vi "4Pi Objective Lock - EMBL-v1.vi"(7 "Calling VI Ref":refnum<vi>) -> ()   [LabVIEW 2016]
uses:
  <vilib>/Utility/miscctls.llb/LVPointTypeDef.ctl
  4Pi Objective Lock Type Defs/4Pi Obj Lock - Notifier Type.ctl
  4Pi Objective Lock Type Defs/4Pi Obj Lock - Actions.ctl
  <vilib>/vision/Image Controls.llb/IMAQ Image.ctl
  4Pi Objective Lock Type Defs/4Pi Obj Lock - Lock Settings.ctl
  Hardware Configuration/Hardware Configuration Controls/Device Type.ctl
  Hardware Configuration/Hardware Configuration Controls/Device Function.ctl
  4Pi Objective Lock Type Defs/4Pi Obj Lock - Camera Settings.ctl
  Device Library/Cameras/Camera Controls/Generic Camera ROI.ctl
  Device Library/Cameras/Camera Controls/Generic Camera Actions.ctl
  Device Library/Stages/Stages Controls/Stage Actions.ctl
  <vilib>/addons/control/pid/pid.llb/PID (DBL).vi
  <vilib>/addons/control/pid/pid.llb/PID (DBL Array).vi
  <vilib>/addons/control/pid/NI_PID_pid.lvlib
  <vilib>/vision/NI_Vision_Development_Module.lvlib
panel:
  out "dz (µm)":dbl format="%.2f"
  in  "Main Tab":T1(tab)
  out "Z Move":bool
  out "XY Move":bool
  out "Measured X Position (px)":dbl=1.0 format="%.3g"
  out "Measured Y Position (px)":dbl=1.0 format="%.3g"
  out "Measured sx/sy":dbl=1.0 format="%.3g"
  out "Target X Position (px)":dbl=1.0 format="%.3g"
  out "Target Y Position (px)":dbl=1.0 format="%.3g"
  out "Target sx/sy":dbl=1.0 format="%.3g"
  out "Z Axis Position (µm)":dbl=1.0 format="%.4g"
  out "Y Axis Position (µm)":dbl=1.0 format="%.2g"
  out "X Axis Position (µm)":dbl=1.0 format="%.2g"
  out "Z Target and Fit Value (µm)":T2(graph)
  in  "Start Lock":bool
  out "Y Target and Fit Position (µm)":T2(graph)
  out "X Target and Fit Position (µm)":T2(graph)
  in  "Restart Lock":bool
  out "Fit Error":bool
  out "Move Limit Error":bool
  out "Target Z (µm)":dbl=1.0 format="%.3g"
  out "Measured Z (µm)":dbl=1.0 format="%.3g"
  in  "pixel size (µm)":dbl=0.01
  in  "X Update Scale Factor":dbl=0.01
  in  "Y Update Scale Factor":dbl=0.01
  in  "Z Update Scale Factor":dbl=0.2
  in  "Sample Z Step No.":u32=2
  in  "Sample Z Step Size (µm)":dbl=2.0
  in  "Update Delay (ms)":i32=10
  in  "D (Derivative)":dbl
  in  "I (Integral)":dbl
  in  "P (Proportional)":dbl=2.0
  in  "Invert Z Axis":bool
  in  "XY Drift Threshold":dbl=0.05
  in  "Abort If Error":bool
  in  "Flip XY Axis":bool
  in  "Invert X Axis":bool=TRUE
  in  "Invert Y Axis":bool=TRUE
  in  "Z Stage Move Limit (µm)":dbl=5.0
  in  "Z Drift Threshold":dbl=0.05
  in  "XY Stage Move Limit (µm)":dbl=1.0
  in  "Frame Accumulations":u16=10
  in  "XY Correction Active":bool=TRUE
  in  "Z Correction Active":bool=TRUE
  in  "Set Camera ROI":bool
  in  "Save Lock Settings":bool
  in  "Quit":bool
  # "Z Drift Settings"
  # "Camera Setup"
  # "XY Drift Settings"
  # "PID Control Values"
  # "General Settings"
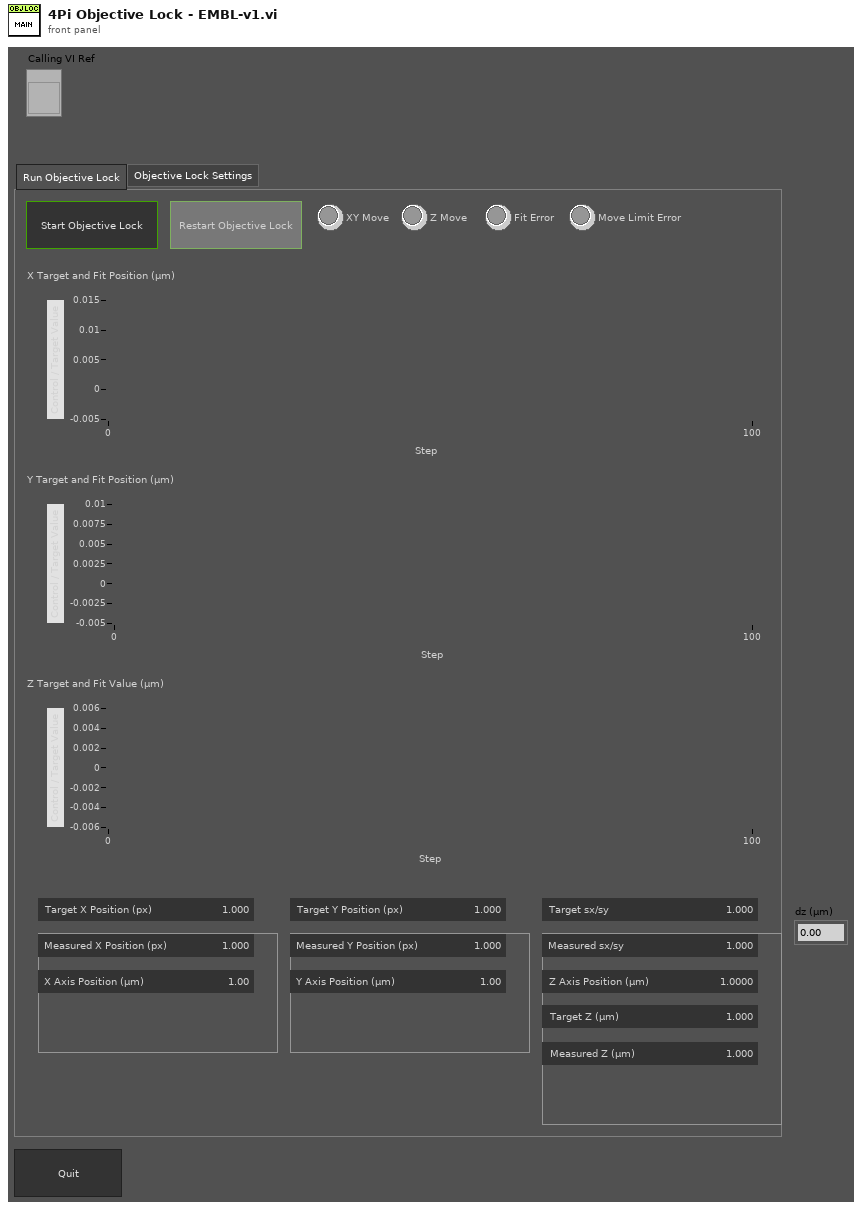
[diagram p1: front panel]
types:
  T1 = enum32{"Run Objective Lock", "Objective Lock Settings"}
  T2 = cluster{"Target 01":dbl, dbl, dbl, "Current 01":dbl, "Stage Pos":dbl}
  T3 = typedef "4Pi Obj Lock - Camera Settings.ctl" = cluster{"Exposure Time (s)":dbl, "H Offset":u16, "V Offset":u16, "H Width":u16, "V Width":u16}
  T4 = typedef "Device Function.ctl" = enum16{"Primary", "Secondary", "Overview", "Wide Field Drift Correction", "642 nm Excitation", "560 nm Excitation", "940 nm Excitation", "546 nm Excitation", "488 nm Excitation", "405 nm Excitation", "Objective Drift Correction", "4Pi Focus Lock", "4Pi Objective Lock", "Objective XY", "Objective Z", "Sample XY", "Sample Coarse Z", "Sample Z", "4Pi Lower", "4Pi Upper", "Mojo", "Adj Cavity", "Line Scanning", "Alert"}
  T5 = typedef "Device Type.ctl" = enum16{"AOTF", "Camera", "Deformable Mirror", "Laser", "Shutter", "Stage", "Waveform", "FPGA", "Email"}
  T6 = typedef "4Pi Obj Lock - Actions.ctl" = enum16{"Idle", "Start Lock", "Restart Lock", "Get Initial Position", "Get Target Z Position", "Get Ref Stack", "Cal Ref FFT", "Move To Init Z", "Get Current Z Position", "Get Current Position", "Check Drift", "Move XYZ", "Move XY", "Move Z", "Update Plots", "Delay", "Abort", "Exit Loop", "Quit"}
  T7 = typedef "4Pi Obj Lock - Lock Settings.ctl" = cluster{"Z Drift Threshold":dbl, "Z Stage Move Limit (µm)":dbl, "XY Drift Threshold":dbl, "XY Stage Move Limit (µm)":dbl, "Frame Accumulations":u16, "Abort If Error":bool, "Flip XY Axis":bool, "Invert X Axis":bool, "Invert Y Axis":bool, "Invert Z Axis":bool, "Z Correction Active":bool, "XY Correction Active":bool, "PID Values":dbl[], "Update Delay (ms)":i32, "Sample Z Step Size (µm)":dbl, "Sample Z Step No.":u32, "Z Update Scale Factor":dbl, "Y Update Scale Factor":dbl, "X Update Scale Factor":dbl}
  T8 = typedef "4Pi Obj Lock - Notifier Type.ctl" = cluster{"Actions":T6, "Z Drift Threshold":dbl, "Z Stage Move Limit (µm)":dbl, "XY Drift Threshold":dbl, "XY Stage Move Limit (µm)":dbl, "Frame Accumulations":u16, "Abort If Error":bool, "Z Correction Active":bool, "XY Correction Active":bool, "PID Values":dbl[], "Running?":bool, "Update Delay (ms)":i32, "Cur Image (SGL)":T9, "Ref Stack (SGL)":T9[], "Sample Z (µm)":dbl[], "Initial Z Position (µm)":dbl, "Z Step Size (µm)":dbl, "Z Step No.":u32, "Ref FFT Stack (CSG)":T9[], "CC Image (SGL) ":T9, "Tmp Image FFT (CSG)":T9[]}
  T9 = typedef "IMAQ Image.ctl" = refnum<image>
  T10 = enum16{"Always On", "Always Off", "Off While Running"}
  T11 = typedef "LVPointTypeDef.ctl" = cluster{"Horizontal":i16, "Vertical":i16}
  T12 = typedef "Image Type" = u32
  T13 = typedef "Generic Camera Actions.ctl" = enum16{"Status", "Live Preview", "Capture", "Abort", "Set Exposure Time (s)", "Get Exposure Time (s)", "Record Settings", "Set ROI", "Get ROI", "Defect Correction On/Off", "Cooler On/Off", "Fan On/Off", "Quit"}
  T14 = typedef "Generic Camera ROI.ctl" = cluster{"H_Offset":u16, "V_Offset":u16, "H_Width":u16, "V_Width":u16}
  T15 = typedef "Stage Actions.ctl" = enum16{"Get Position", "MVR", "MOVE", "HALT", "ONTARGET", "ERROR", "REFERENCE", "INIT", "VELOCITY", "STATUS", "EXIT", "HOME", "ZEROPOS", "NANOPOS", "ANALOG", "QUIT"}
  T16 = enum32{"Invalid", "Standard", "Closed", "Hidden", "Minimized", "Maximized"}
  T17 = cluster{"Target 01":dbl, dbl, dbl, "Current 01":dbl, "Stage Pos":dbl}[]
  T18 = typedef "Stage Status.ctl" = enum16{"Error", "Abort", "Busy", "On Target"}
  T19 = typedef "2D Gaussian - Best Fit Parameters.ctl" = cluster{"Amplitude":dbl, "X Position":dbl, "Y Position":dbl, "X Width":dbl, "Y Width":dbl, "Offset":dbl}
  T20 = cluster{"PID Values[0]":dbl, "PID Values[1]":dbl, "PID Values[2]":dbl}
  T21 = cluster{"PID Values[0]":dbl, "PID Values[1]":dbl, "PID Values[2]":dbl}[]
  T22 = typedef "LVRectTypeDef.ctl" = cluster{"Left":i16, "Top":i16, "Right":i16, "Bottom":i16}
  T23 = typedef "LVBoundsTypeDef.ctl" = cluster{"Width":u32, "Height":u32}
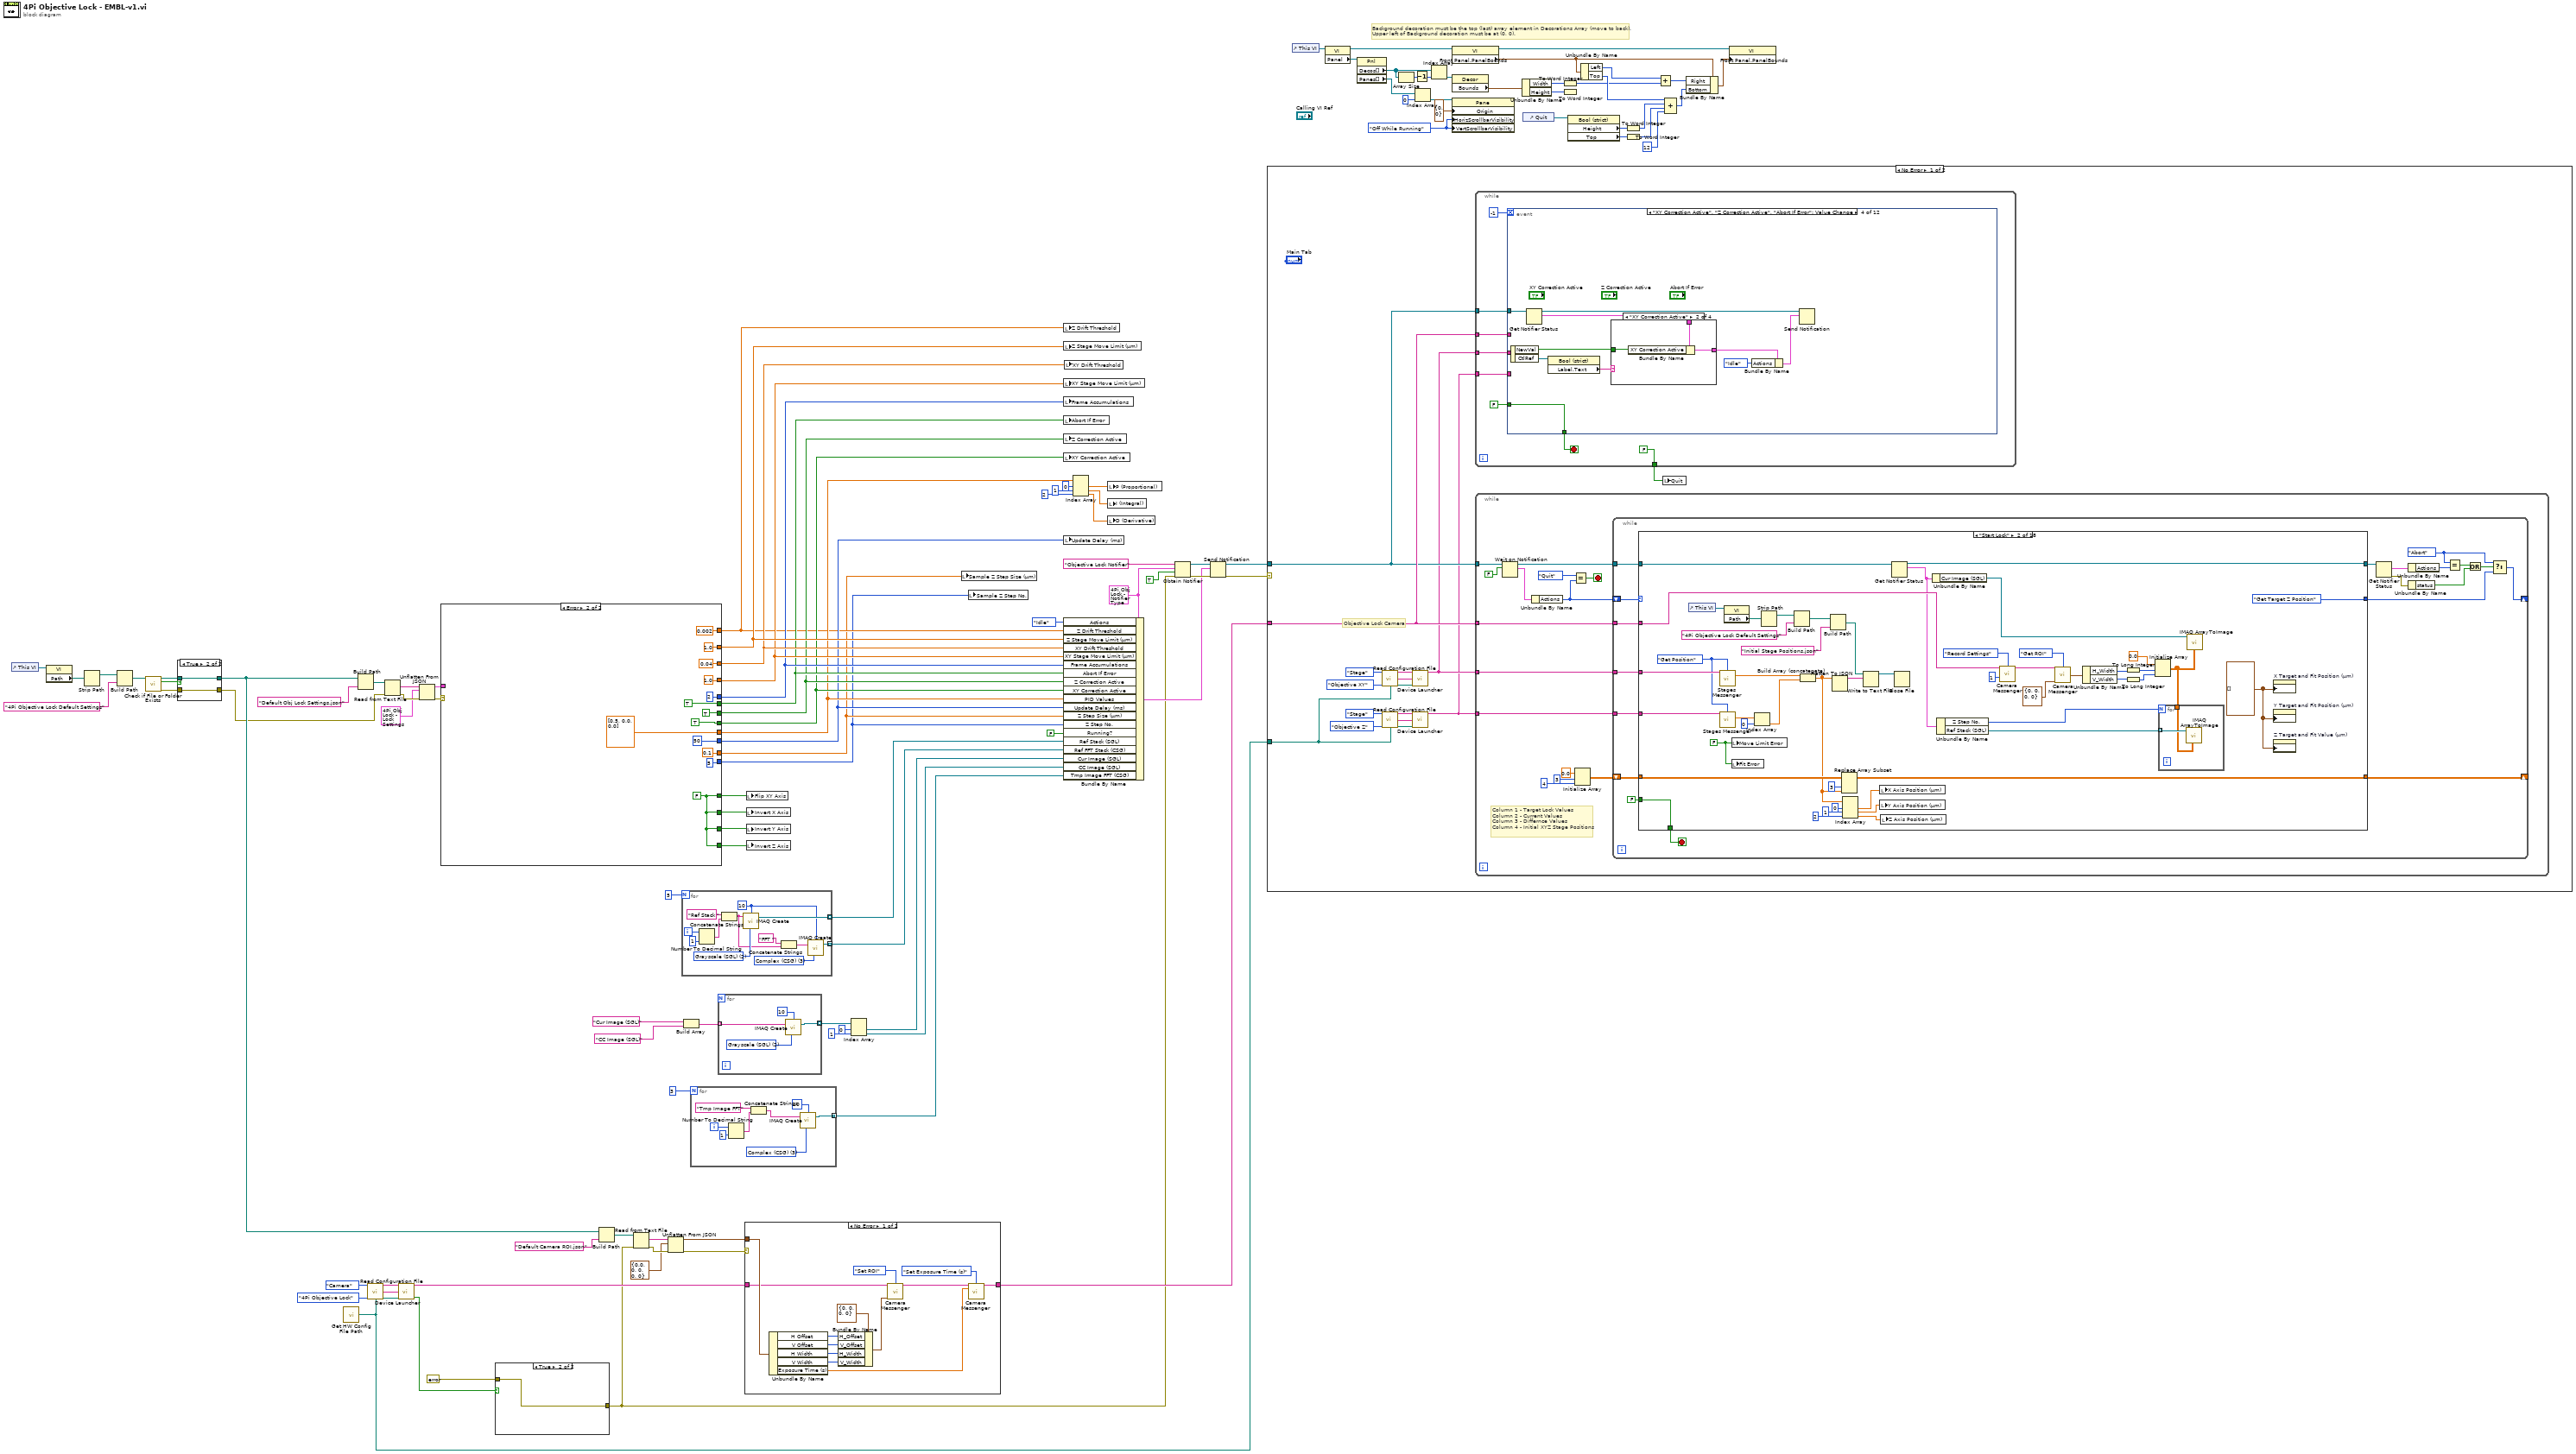
[diagram p0: block diagram]
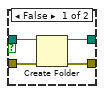
[diagram p2: hidden frame]
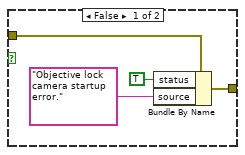
[diagram p3: hidden frame]
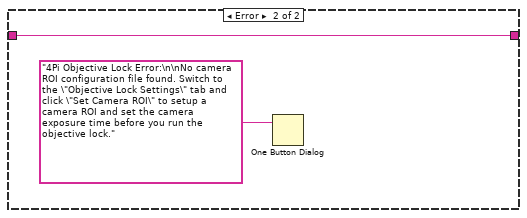
[diagram p4: hidden frame]
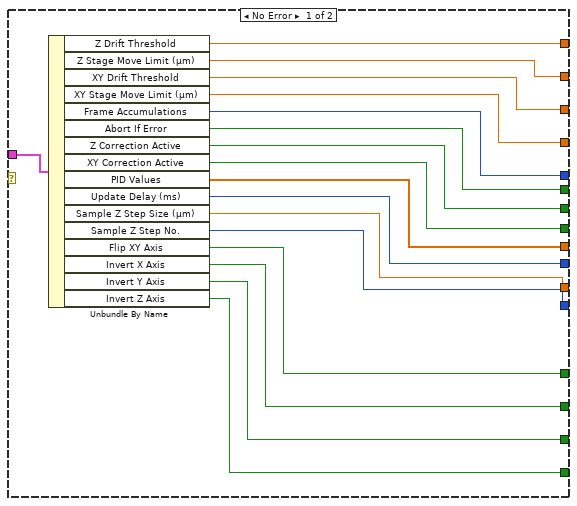
[diagram p5: hidden frame]
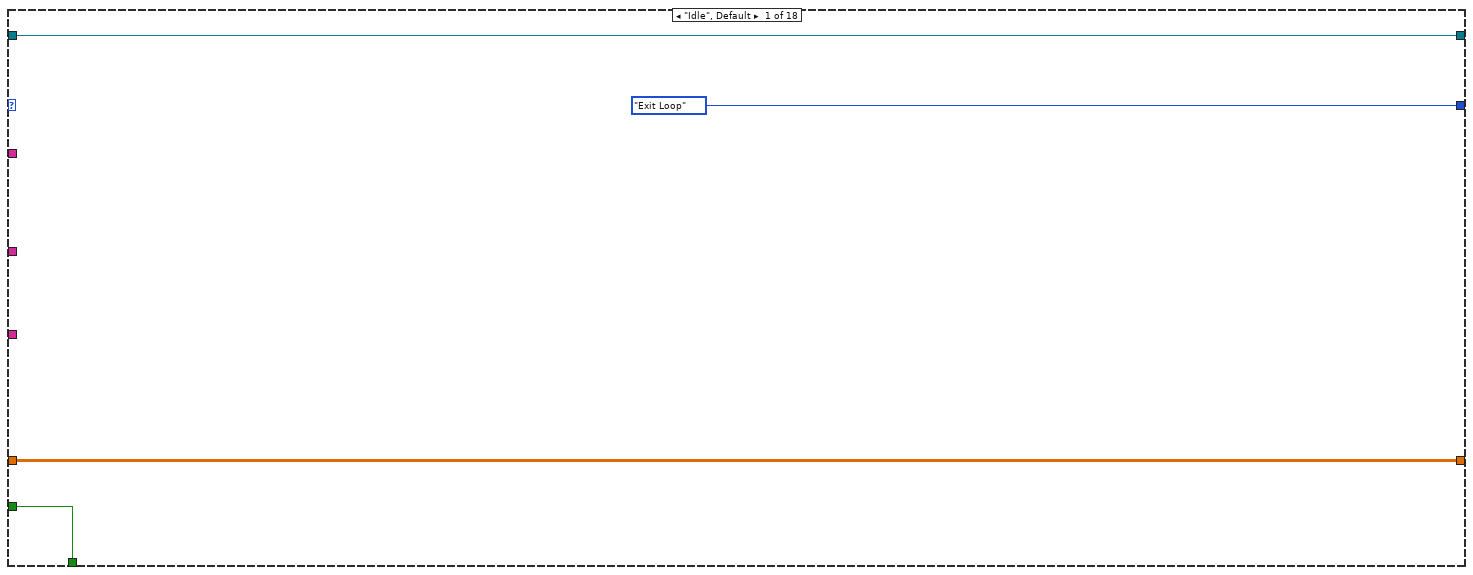
[diagram p6: hidden frame]
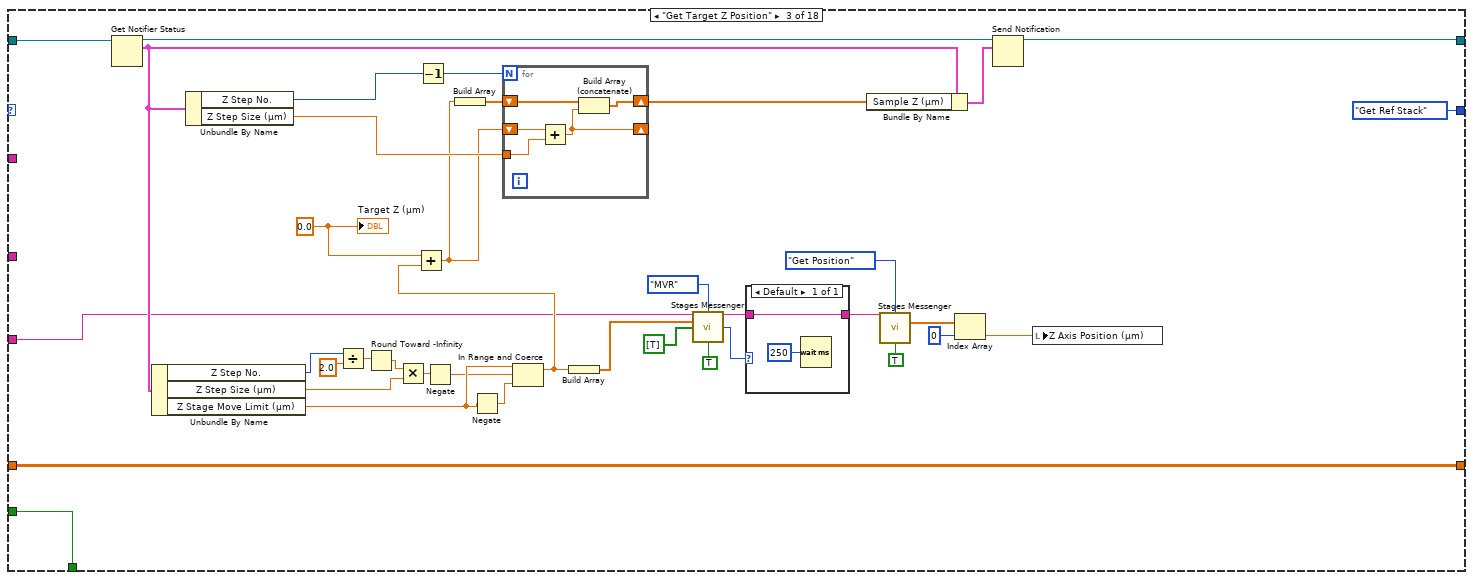
[diagram p7: hidden frame]
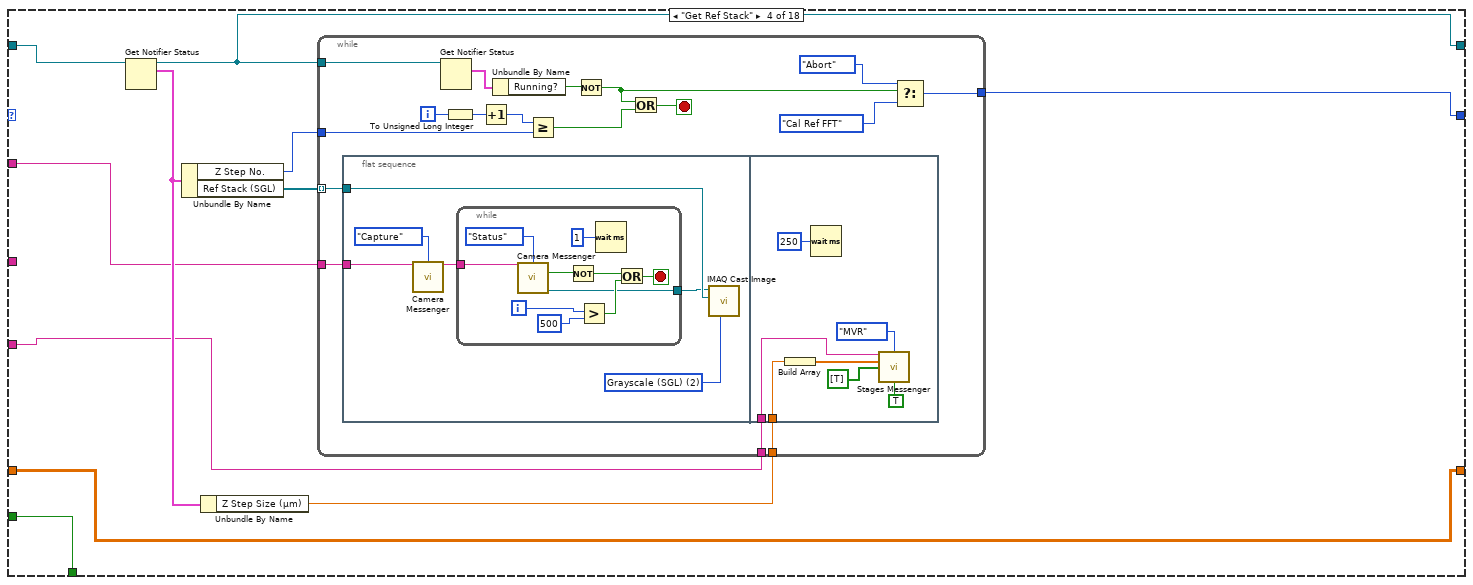
[diagram p8: hidden frame]
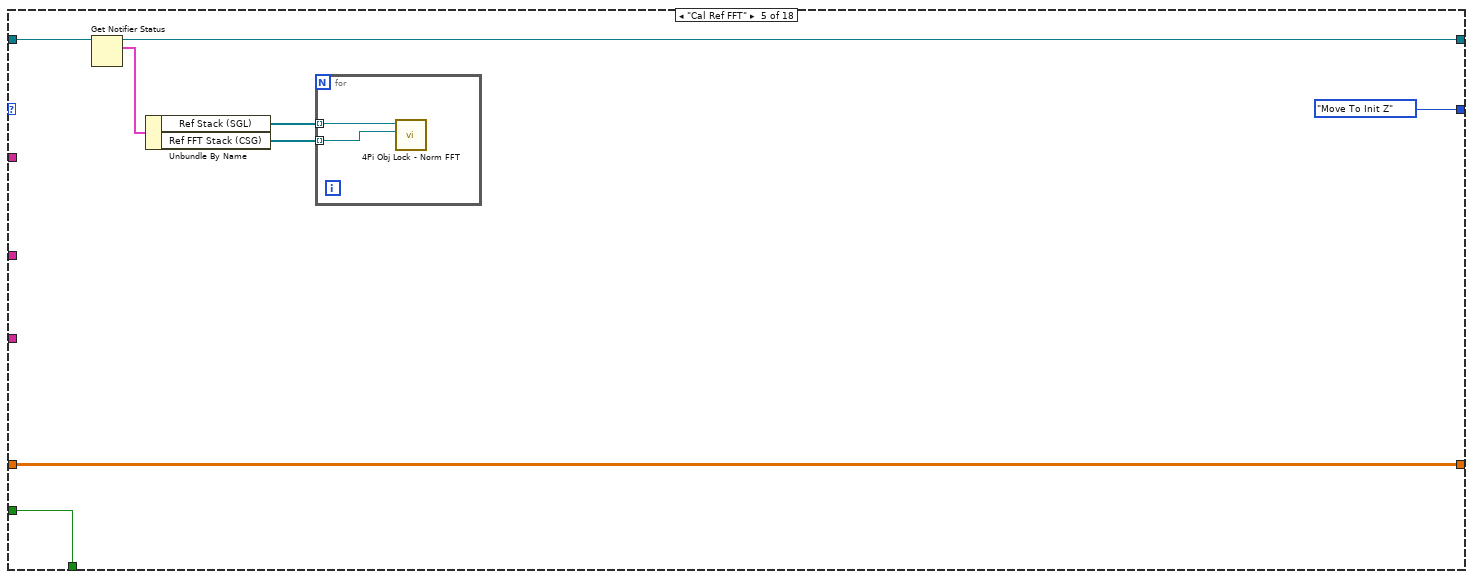
[diagram p9: hidden frame]
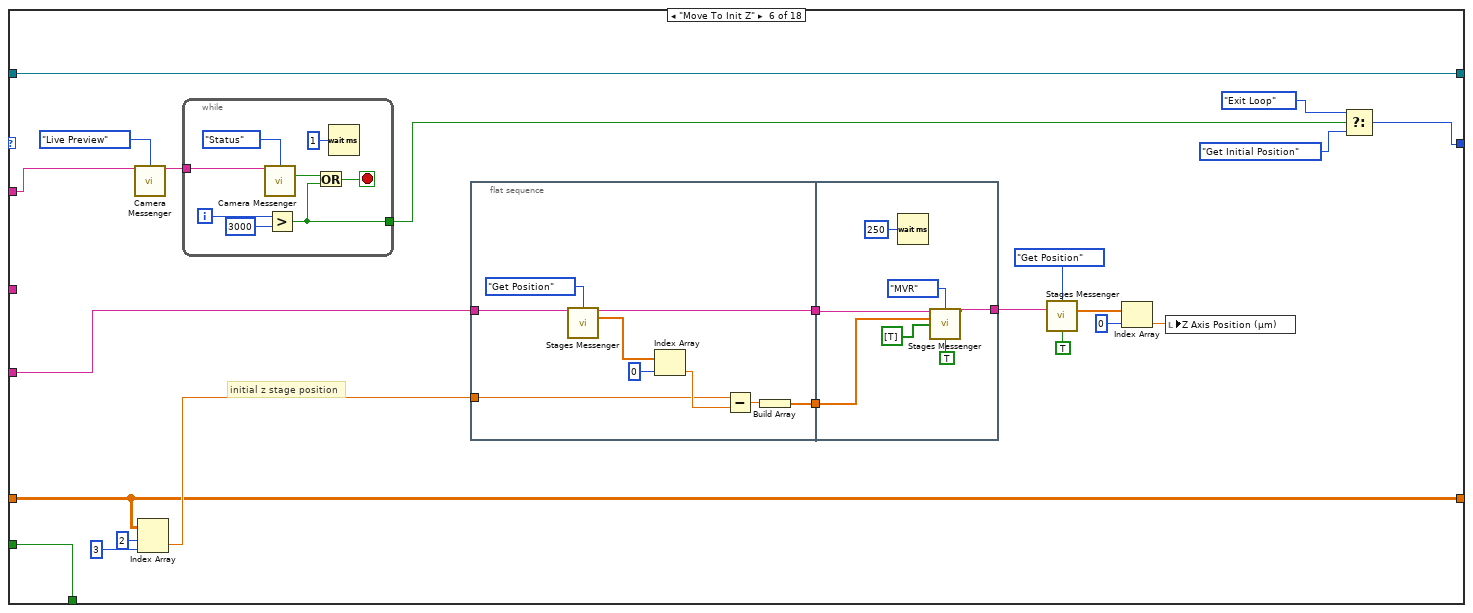
[diagram p10: hidden frame]
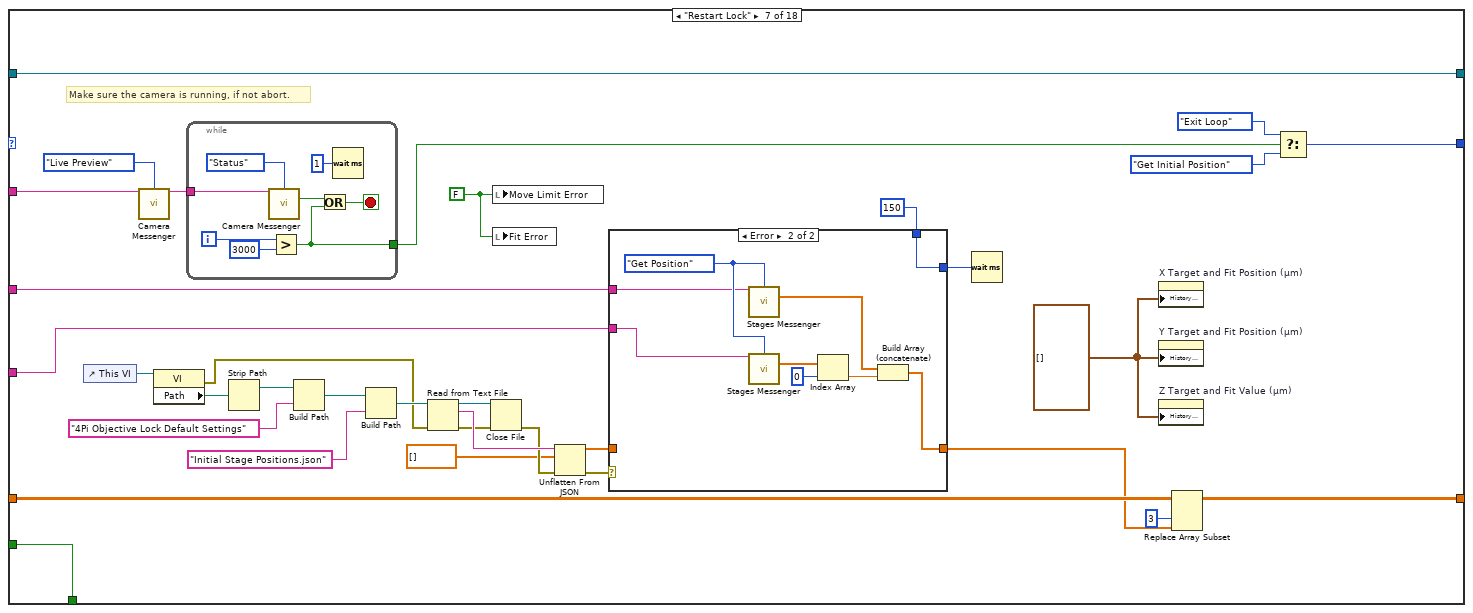
[diagram p11: hidden frame]
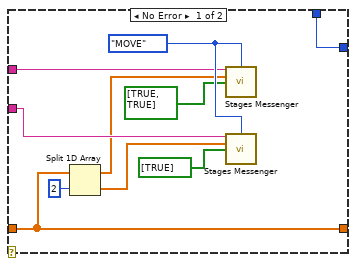
[diagram p12: hidden frame]
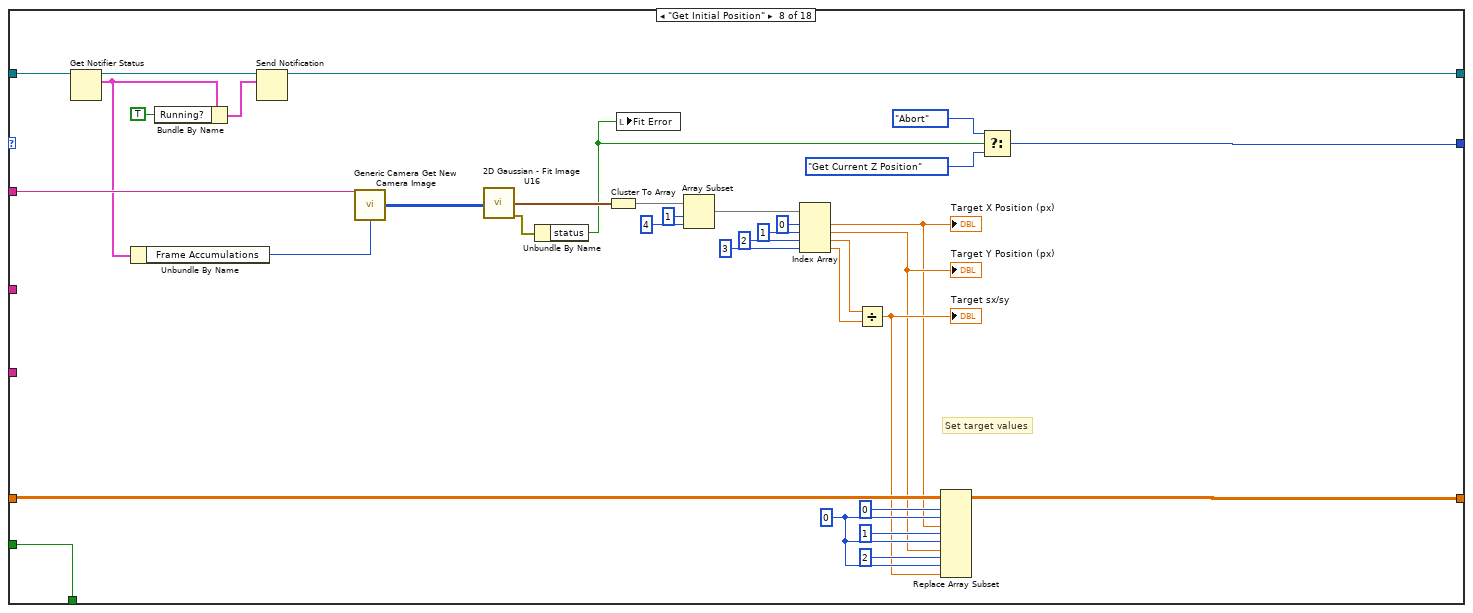
[diagram p13: hidden frame]
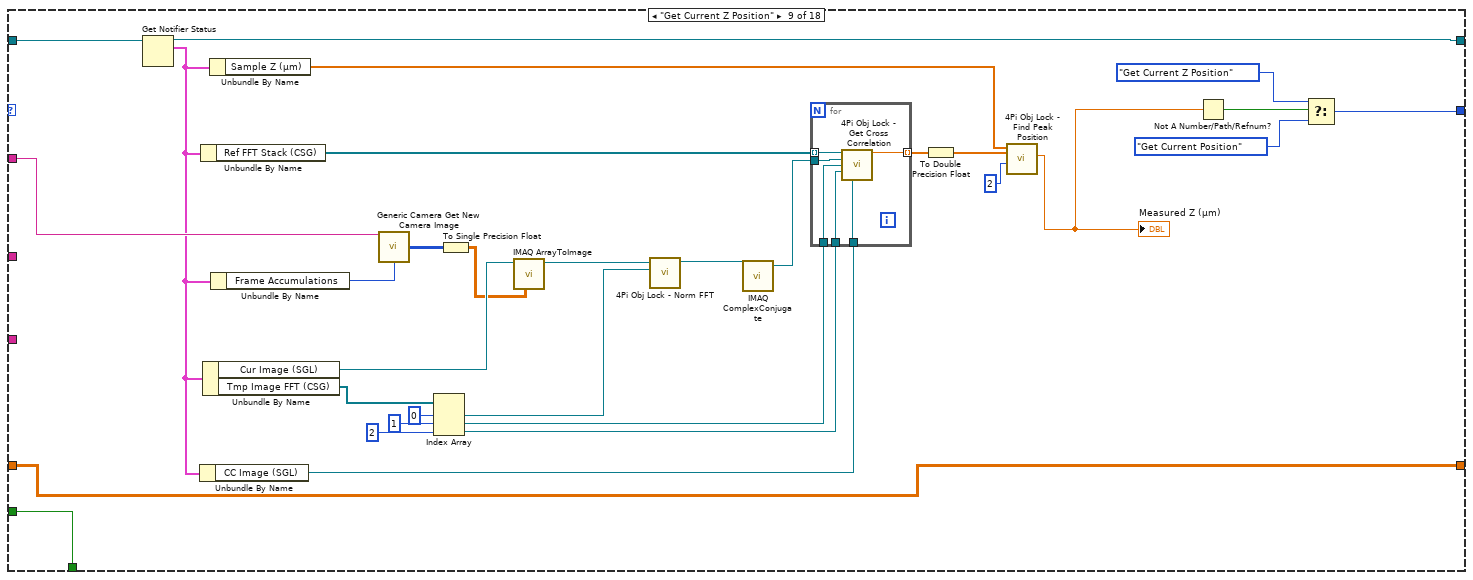
[diagram p14: hidden frame]
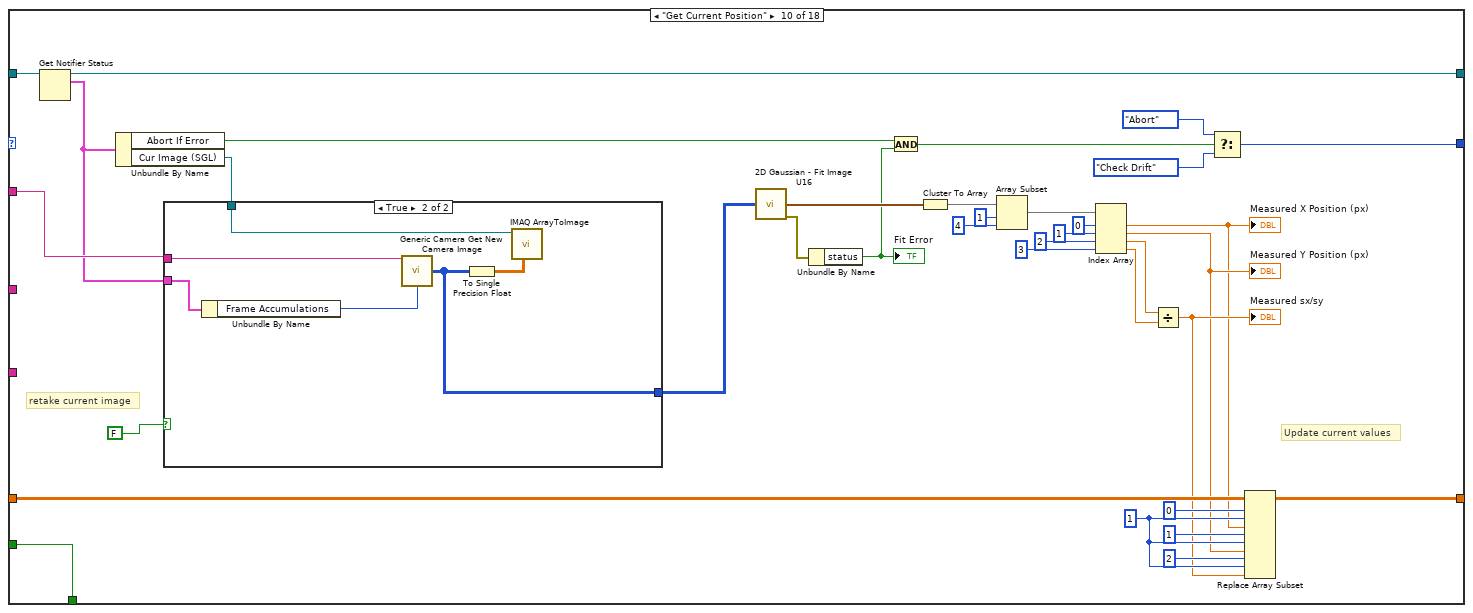
[diagram p15: hidden frame]
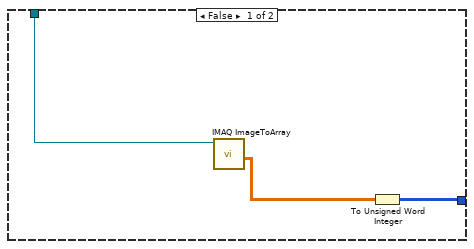
[diagram p16: hidden frame]
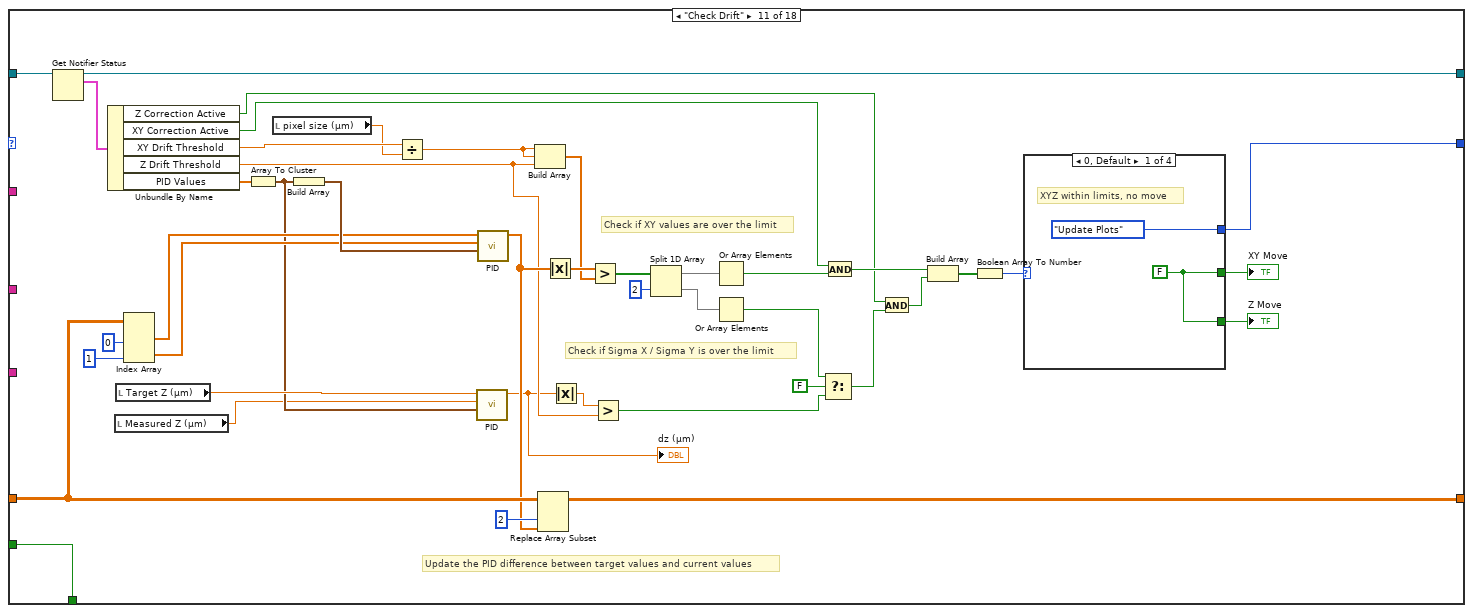
[diagram p17: hidden frame]
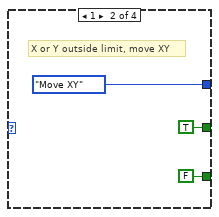
[diagram p18: hidden frame]
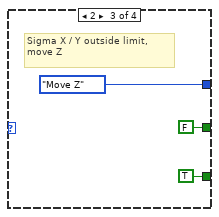
[diagram p19: hidden frame]
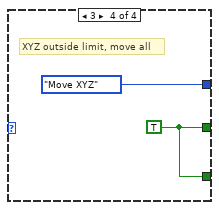
[diagram p20: hidden frame]
diagram:
  w75 = T8 {"Actions"=enum."Idle", "Z Drift Threshold"=0.05, "Z Stage Move Limit (µm)"=1.0, "XY Drift Threshold"=0.05, "XY Stage Move Limit (µm)"=1.0, "Frame Accumulations"=10, "Abort If Error"=FALSE, "Z Correction Active"=FALSE, "XY Correction Active"=FALSE, "PID Values"=[], "Running?"=FALSE, "Update Delay (ms)"=0, "Cur Image (SGL)"=refnum, "Ref Stack (SGL)"=[], "Sample Z (µm)"=[], "Initial Z Position (µm)"=0.0, "Z Step Size (µm)"=2.0, "Z Step No."=2, "Ref FFT Stack (CSG)"=[], "CC Image (SGL) "=refnum, "Tmp Image FFT (CSG)"=[]} ("4Pi Obj Lock")
  w92 = T10."Off While Running" ("Vertical Scrollbar Visibility")
  # "Background decoration must be the top (last) array element in Decorations Array (move to back).\nUpper left of Background decoration must be at (0, 0)."
  n1 = control-ref of="This VI"() -> (w63:refnum<vi>)
  n2 = property class="VI"(reference=w63) -> ("Path"=w45:path)  [unwired: 1 in, 2 out]
  n3 = Strip Path(path=w45) -> (stripped path=w44:path)  [unwired: 1 out]
  n4 = Build Path(base path=w44, name or relative path="4Pi Objective Lock Default Settings") -> (appended path=w21:path)
  n5 = call <vilib>:"Check if File or Folder Exists.vi"("path"=w21) -> ("error out"=w17:errorcluster, "file or folder exists?"=w20:bool, "dup path"=w19:path)  [unwired: 8 in]
  n6 = case shown="True" w20 {
    tunnel: w19 -> [w113 w115]
    tunnel: [w112 w115] -> w18
    tunnel: w17 -> [w111 w114]
    tunnel: [w110 w114] -> w16
    frame False {
      n7 = Create Folder(path (use dialog)=w113, error in=w111) -> (created path=w112:path, error out=w110:errorcluster)  [unwired: 1 in, 1 out]
    }
    frame True {
    }
  }
  n8 = call "Get HW Config File Path.vi"() -> ("File Path"=w53:path)  [unwired: 14 in, 1 out]
  n9 = Build Path(base path=w18, name or relative path="Default Obj Lock Settings.json") -> (appended path=w72:path)
  n10 = call "Read Configuration File.vi"("Device Type"=Device_Type."Camera", "Device Function"=Device_Function."4Pi Objective Lock", "Config File Path"=w53) -> ("Unique Notifier Name"=w60:string, "Device Ports/IDs/Channels"=w62:string[], "Device Engine Path"=w61:path)  [unwired: 9 in, 1 out]
  n11 = Read from Text File(file (use dialog)=w72, error in=w16) -> (text=w71:string, error out=w70:errorcluster)  [unwired: 2 in, 2 out]
  n12 = call "Device Launcher.vi"("Notifier Name"=w60, "Device Ports/IDs/Channels"=w62, "Device Engine Path"=w61) -> ("Notifier Name"=w51:string, "Running?"=w57:bool)  [unwired: 11 in]
  n13 = Unflatten From JSON(JSON string=w71, type and defaults=T7 {"Z Drift Threshold"=0.05, "Z Stage Move Limit (µm)"=1.0, "XY Drift Threshold"=0.05, "XY Stage Move Limit (µm)"=1.0, "Frame Accumulations"=10, "Abort If Error"=FALSE, "Flip XY Axis"=FALSE, "Invert X Axis"=FALSE, "Invert Y Axis"=FALSE, "Invert Z Axis"=FALSE, "Z Correction Active"=TRUE, "XY Correction Active"=TRUE, "PID Values"=[], "Update Delay (ms)"=0, "Sample Z Step Size (µm)"=2.0, "Sample Z Step No."=2, "Z Update Scale Factor"=2.0, "Y Update Scale Factor"=2.0, "X Update Scale Factor"=2.0} ("Lock Settings"), error in (no error)=w70) -> (value=w67:T7, error out=w68:errorcluster)  [unwired: 4 in]
  n14 = case shown="Error" w68 {
    tunnel: [w131 0.002 ("Z Drift Threshold")] -> w22
    tunnel: [w130 1.0 ("Z Stage Move Limit (µm)")] -> w37
    tunnel: [w128 0.04 ("XY Drift Threshold")] -> w36
    tunnel: [w129 1.0 ("XY Stage Move Limit (µm)")] -> w35
    tunnel: [w127 u16 2 ("Frame Accumulations")] -> w34
    tunnel: [w126 TRUE ("Abort If Error")] -> w33
    tunnel: w67 -> [w132 _]
    tunnel: [w125 TRUE ("Z Correction Active")] -> w32
    tunnel: [w124 TRUE ("XY Correction Active")] -> w31
    tunnel: [w123 dbl[] [0.5, 0.0, 0.0] ("PID Values")] -> w30
    tunnel: [w122 u16 50 ("Update Delay (ms)")] -> w23
    tunnel: [w121 w135] -> w39
    tunnel: [w120 w135] -> w40
    tunnel: [w119 w135] -> w41
    tunnel: [w118 w135] -> w42
    tunnel: [w117 0.1 ("Sample Z Step Size (µm)")] -> w2
    tunnel: [w116 u32 5 ("Sample Z Step No.")] -> w1
    frame No Error {
      n15 = Unbundle By Name(w132) -> ("Z Drift Threshold"=w131:dbl, "Z Stage Move Limit (µm)"=w130:dbl, "XY Drift Threshold"=w128:dbl, "XY Stage Move Limit (µm)"=w129:dbl, "Frame Accumulations"=w127:u16, "Abort If Error"=w126:bool, "Z Correction Active"=w125:bool, "XY Correction Active"=w124:bool, "PID Values"=w123:dbl[], "Update Delay (ms)"=w122:i32, "Sample Z Step Size (µm)"=w117:dbl, "Sample Z Step No."=w116:u32, "Flip XY Axis"=w118:bool, "Invert X Axis"=w119:bool, "Invert Y Axis"=w120:bool, "Invert Z Axis"=w121:bool)
    }
    frame Error {
      w135 = FALSE ("Flip XY Axis")
    }
  }
  n16 = case shown="True" w57 {
    tunnel: errorcluster {"status"=FALSE, "code"=0, "source"=""} ("Error") -> [w149 w150]
    tunnel: [w146 w150] -> w43
    frame False {
      n17 = Bundle By Name(cluster=w149, "status"=TRUE, "source"="Objective lock camera startup error." ("name or relative path")) -> (w146:errorcluster)
    }
    frame True {
    }
  }
  n18 = Build Path(base path=w18, name or relative path="Default Camera ROI.json") -> (appended path=w47:path)
  n19 = Read from Text File(file (use dialog)=w47, error in=w43) -> (text=w65:string, error out=w64:errorcluster)  [unwired: 2 in, 2 out]
  n20 = Unflatten From JSON(JSON string=w65, type and defaults=T3 {"Exposure Time (s)"=0.0, "H Offset"=0, "V Offset"=0, "H Width"=0, "V Width"=0} ("Camera Settings"), error in (no error)=w64) -> (value=w50:T3, error out=w55:errorcluster)  [unwired: 4 in]
  n21 = for {
    N: 5 -> [_]
    tunnel: [w162] -> w14 mode=indexing
    tunnel: [w151] -> w13 mode=indexing
    i -> [w161]
    w156 = T12 3 items=["Grayscale (U8)", "Grayscale (I16)", "Grayscale (SGL)", "Complex (CSG)", "RGB (U32)", "HSL (U32)", "RGB (U64)", "Grayscale (U16)"] ("Image Type")
    w157 = T12 2 items=["Grayscale (U8)", "Grayscale (I16)", "Grayscale (SGL)", "Complex (CSG)", "RGB (U32)", "HSL (U32)", "RGB (U64)", "Grayscale (U16)"] ("Image Type")
    w153 = 10 ("Border Size")
    n22 = Number To Decimal String(number=w161, width (-)=i16 1) -> (decimal integer string=w159:string)
    n23 = Concatenate Strings("Ref Stack " ("string"), w159) -> (w152:string)
    n24 = call "IMAQ Create"("Border Size"=w153, "Image Name"=w152, "Image Type"=w157) -> ("New Image"=w162:T9)  [unwired: 2 in, 1 out]
    n25 = Concatenate Strings("FFT " ("string"), w152) -> (w155:string)
    n26 = call "IMAQ Create"("Border Size"=w153, "Image Name"=w155, "Image Type"=w156) -> ("New Image"=w151:T9)  [unwired: 2 in, 1 out]
  }
  n27 = Build Array("Cur Image (SGL)" ("Image Name"), "CC Image (SGL)" ("Image Name")) -> (w8:string[])
  n28 = for {
    N: 3 -> [_]
    tunnel: [w168] -> w3 mode=indexing
    i -> [w164]
    w169 = T12 3 items=["Grayscale (U8)", "Grayscale (I16)", "Grayscale (SGL)", "Complex (CSG)", "RGB (U32)", "HSL (U32)", "RGB (U64)", "Grayscale (U16)"] ("Image Type")
    n29 = Number To Decimal String(number=w164, width (-)=i16 1) -> (decimal integer string=w167:string)
    n30 = Concatenate Strings("Tmp Image FFT" ("Image Name"), w167) -> (w163:string)
    n31 = call "IMAQ Create"("Border Size"=10, "Image Name"=w163, "Image Type"=w169) -> ("New Image"=w168:T9)  [unwired: 2 in, 1 out]
  }
  n32 = for {
    tunnel: w8 -> [w172] mode=indexing
    tunnel: [w171] -> w7 mode=indexing
    w173 = T12 2 items=["Grayscale (U8)", "Grayscale (I16)", "Grayscale (SGL)", "Complex (CSG)", "RGB (U32)", "HSL (U32)", "RGB (U64)", "Grayscale (U16)"] ("Image Type")
    n33 = call "IMAQ Create"("Border Size"=10, "Image Name"=w172, "Image Type"=w173) -> ("New Image"=w171:T9)  [unwired: 2 in, 1 out]
  }
  n34 = case shown="No Error" w55 {
    tunnel: w51 -> [w178 w189]
    tunnel: w50 -> [w187 _]
    tunnel: [w175 w189] -> w49
    frame No Error {
      n35 = Unbundle By Name(w187) -> ("H Offset"=w182:u16, "V Offset"=w183:u16, "H Width"=w184:u16, "V Width"=w185:u16, "Exposure Time (s)"=w177:dbl)
      n36 = Bundle By Name(cluster=T14 {"H_Offset"=0, "V_Offset"=0, "H_Width"=0, "V_Width"=0} ("General Camera ROI"), "H_Offset"=w182, "V_Offset"=w183, "H_Width"=w184, "V_Width"=w185) -> (w181:T14)
      n37 = call "Camera Messenger.vi"("Notifier Name"=w178, "General Camera Actions"=Generic_Camera_Actions."Set ROI", "Camera ROI"=w181) -> ("Notifier Name Dup"=w176:string)  [unwired: 7 in, 5 out]
      n38 = call "Camera Messenger.vi"("Notifier Name"=w176, "General Camera Actions"=Generic_Camera_Actions."Set Exposure Time (s)", "Exposure Time (s)"=w177) -> ("Notifier Name Dup"=w175:string)  [unwired: 7 in, 5 out]
    }
    frame Error {
      n39 = One Button Dialog(message="4Pi Objective Lock Error:\n\nNo camera ROI configuration file found. Switch to the \"Objective Lock Settings\" tab and click \"Set Camera ROI\" to setup a camera ROI and set the camera exposure time before you run the objective lock.") -> ()  [unwired: 1 in, 1 out]
    }
  }
  n40 = local write "Flip XY Axis"(w42) -> ()
  n41 = local write "Invert X Axis"(w41) -> ()
  n42 = local write "Invert Y Axis"(w40) -> ()
  n43 = local write "Invert Z Axis"(w39) -> ()
  n44 = Index Array(array=w7, index #1=0 ("index"), index #2=1 ("index")) -> (element #1=w6:T9, element #2=w5:T9)
  n45 = local write "Sample Z Step Size (µm)"(w2) -> ()
  n46 = local write "Sample Z Step No."(w1) -> ()
  n47 = Bundle By Name(cluster=w75, "Actions"=4Pi_Obj_Lock_-_Actions."Idle", "Z Drift Threshold"=w22, "Z Stage Move Limit (µm)"=w37, "XY Drift Threshold"=w36, "XY Stage Move Limit (µm)"=w35, "Frame Accumulations"=w34, "Abort If Error"=w33, "Z Correction Active"=w32, "XY Correction Active"=w31, "PID Values"=w30, "Update Delay (ms)"=w23, "Z Step Size (µm)"=w2, "Z Step No."=w1, "Running?"=FALSE ("Obj Lock Active?"), "Ref Stack (SGL)"=w14, "Ref FFT Stack (CSG)"=w13, "Cur Image (SGL)"=w6, "CC Image (SGL)"=w5, "Tmp Image FFT (CSG)"=w3) -> (w74:T8)
  n48 = local write "Z Drift Threshold"(w22) -> ()
  n49 = local write "Z Stage Move Limit (µm)"(w37) -> ()
  n50 = local write "XY Stage Move Limit (µm)"(w35) -> ()
  n51 = local write "Frame Accumulations"(w34) -> ()
  n52 = local write "Abort If Error"(w33) -> ()
  n53 = local write "Z Correction Active"(w32) -> ()
  n54 = local write "XY Correction Active"(w31) -> ()
  n55 = local write "Update Delay (ms)"(w23) -> ()
  n56 = local write "XY Drift Threshold"(w36) -> ()
  n57 = Index Array(array=w30, index #1=0 ("index"), index #2=1 ("index"), index #3=2 ("index")) -> (element #1=w26:dbl, element #2=w24:dbl, element #3=w25:dbl)
  n58 = local write "P (Proportional)"(w26) -> ()
  n59 = local write "I (Integral)"(w24) -> ()
  n60 = local write "D (Derivative)"(w25) -> ()
  n61 = Obtain Notifier(name (unnamed)="Objective Lock Notifier", notification data type=w75, create if not found? (T)=TRUE, error in (no error)=w43) -> (notifier out=w77:refnum<notifier>, error out=w78:errorcluster)  [unwired: 1 out]
  n62 = Send Notification(notification=w74, notifier=w77, error in (no error)=w78) -> (notifier out=w76:refnum<notifier>, error out=w54:errorcluster)
  n63 = case shown="No Error" w54 {
    tunnel: w53 -> [w194 _]
    tunnel: w76 -> [w192 _]
    tunnel: w49 -> [w193 _]
    frame No Error {
      # "Objective Lock Camera"
      n64 = call "Read Configuration File.vi"("Device Type"=Device_Type."Stage", "Device Function"=Device_Function."Objective XY", "Config File Path"=w194) -> ("Unique Notifier Name"=w202:string, "Device Ports/IDs/Channels"=w200:string[], "Device Engine Path"=w201:path)  [unwired: 9 in, 1 out]
      n65 = call "Read Configuration File.vi"("Device Type"=Device_Type."Stage", "Device Function"=Device_Function."Objective Z", "Config File Path"=w194) -> ("Unique Notifier Name"=w197:string, "Device Ports/IDs/Channels"=w199:string[], "Device Engine Path"=w198:path)  [unwired: 9 in, 1 out]
      n66 = call "Device Launcher.vi"("Notifier Name"=w202, "Device Ports/IDs/Channels"=w200, "Device Engine Path"=w201) -> ("Notifier Name"=w191:string)  [unwired: 11 in, 1 out]
      n67 = call "Device Launcher.vi"("Notifier Name"=w197, "Device Ports/IDs/Channels"=w199, "Device Engine Path"=w198) -> ("Notifier Name"=w190:string)  [unwired: 11 in, 1 out]
      n68 = while {
        tunnel: [FALSE] -> w205
        tunnel: w193 -> [w898]
        tunnel: w192 -> [w897]
        tunnel: w191 -> [w896]
        tunnel: w190 -> [w895]
        stop <- w900 stop-if-true
        n69 = event shown="[3] \"XY Correction Active\", \"Z Correction Active\", \"Abort If Error\": Value Change" {
          selector: _ -> [_ _ _ _ _ _ _ _ _ _ _ _]
          dyn-events: _ -> [_ _ _ _ _ _ _ _ _ _ _ _]
          timeout: -1 -> [_ _ _ _ _ _ _ _ _ _ _ _]
          tunnel: FALSE -> [w903 w907 w910 w920 w940 w975 w1002 w1009 w1038 w1048 w1055 _]
          tunnel: [w903 w907 w910 w920 w940 w975 w1002 w1009 w1038 w1048 w1055 w1065] -> w900
          tunnel: w898 -> [_ _ w909 _ _ _ _ _ _ _ _ _]
          tunnel: w897 -> [_ _ _ w919 w937 w978 w1001 w1008 w1037 w1047 w1054 w1060]
          tunnel: w896 -> [_ _ _ _ _ _ _ _ _ _ _ _]
          tunnel: w895 -> [_ _ _ _ _ _ _ _ _ _ _ _]
          event Timeout {
            n70 = event-data() -> ()  [unwired: 1 in, 1 out]
          }
          event Application Instance Close? {
            n71 = event-data() -> ()  [unwired: 1 in, 1 out]
            n72 = control-ref of="This VI"() -> (w904:refnum<vi>)
            n73 = invoke class="VI" method="FP.Open"(reference=w904, "Activate"=TRUE ("Activate?"), "State"=T16."Standard") -> ()  [unwired: 2 in, 5 out]
            n74 = event-data("Discard?"=TRUE) -> ()  [unwired: 1 in, 1 out]
          }
          event "Set Camera ROI": Value Change {
            n75 = event-data() -> ()  [unwired: 1 in, 2 out]
            n76 = call "4Pi Obj Lock - Setup Camera.vi"("Camera Notifier Name"=w909) -> ()  [unwired: 14 in, 1 out]
          }
          event "XY Correction Active", "Z Correction Active", "Abort If Error": Value Change {
            n77 = event-data() -> ("NewVal"=w915:bool, "CtlRef"=w918:refnum<vi>)  [unwired: 1 in]
            n78 = Get Notifier Status(notifier=w919) -> (notifier out=w917:refnum<notifier>, current notification=w914:T8)  [unwired: 1 in, 3 out]
            n79 = property class="Bool (strict)"(reference=w918) -> ("Label.Text"=w916:string)  [unwired: 1 in, 2 out]
            n80 = case shown="\"XY Correction Active\"" w916 {
              tunnel: w915 -> [_ w923 w926 w929]
              tunnel: w914 -> [w921 w924 w927 w930]
              tunnel: [w921 w922 w925 w928] -> w913
              frame Default {
              }
              frame "XY Correction Active" {
                n81 = Bundle By Name(cluster=w924, "XY Correction Active"=w923) -> (w922:T8)
              }
              frame "Z Correction Active" {
                n82 = Bundle By Name(cluster=w927, "Z Correction Active"=w926) -> (w925:T8)
              }
              frame "Abort If Error" {
                n83 = Bundle By Name(cluster=w930, "Abort If Error"=w929) -> (w928:T8)
              }
            }
            n84 = Bundle By Name(cluster=w913, "Actions"=4Pi_Obj_Lock_-_Actions."Idle") -> (w911:T8)
            n85 = Send Notification(notification=w911, notifier=w917) -> ()  [unwired: 1 in, 2 out]
          }
          event "Z Drift Threshold", "Z Stage Move Limit (µm)", "XY Drift Threshold", "XY Stage Move Limit (µm)", "P (Proportional)", "I (Integral)", "D (Derivative)", "Sample Z Step Size (µm)": Value Change {
            n86 = event-data() -> ("NewVal"=w935:dbl, "CtlRef"=w936:refnum<vi>)  [unwired: 1 in]
            n87 = Get Notifier Status(notifier=w937) -> (notifier out=w934:refnum<notifier>, current notification=w938:T8)  [unwired: 1 in, 3 out]
            n88 = property class="DigNum (strict)"(reference=w936) -> ("Label.Text"=w939:string)  [unwired: 1 in, 2 out]
            n89 = case shown="\"Sample Z Step Size (µm)\"" w939 {
              tunnel: w935 -> [_ w943 w946 w949 w952 w957 w963 w969 w973]
              tunnel: w938 -> [w941 w944 w947 w950 w953 w956 w962 w968 w974]
              tunnel: [w941 w942 w945 w948 w951 w954 w960 w966 w972] -> w932
              frame Default {
              }
              frame "Z Drift Threshold" {
                n90 = Bundle By Name(cluster=w944, "Z Drift Threshold"=w943) -> (w942:T8)
              }
              frame "Z Stage Move Limit (µm)" {
                n91 = Bundle By Name(cluster=w947, "Z Stage Move Limit (µm)"=w946) -> (w945:T8)
              }
              frame "XY Drift Threshold" {
                n92 = Bundle By Name(cluster=w950, "XY Drift Threshold"=w949) -> (w948:T8)
              }
              frame "XY Stage Move Limit (µm)" {
                n93 = Bundle By Name(cluster=w953, "XY Stage Move Limit (µm)"=w952) -> (w951:T8)
              }
              frame "P (Proportional)" {
                n94 = Unbundle By Name(w956) -> ("PID Values"=w959:dbl[])
                n95 = Replace Array Subset(array=w959, new element=w957, index=0) -> (w955:dbl[])
                n96 = Bundle By Name(cluster=w956, "PID Values"=w955) -> (w954:T8)
              }
              frame "I (Integral)" {
                n97 = Unbundle By Name(w962) -> ("PID Values"=w965:dbl[])
                n98 = Replace Array Subset(array=w965, new element=w963, index=1) -> (w961:dbl[])
                n99 = Bundle By Name(cluster=w962, "PID Values"=w961) -> (w960:T8)
              }
              frame "D (Derivative)" {
                n100 = Unbundle By Name(w968) -> ("PID Values"=w971:dbl[])
                n101 = Replace Array Subset(array=w971, new element=w969, index=2) -> (w967:dbl[])
                n102 = Bundle By Name(cluster=w968, "PID Values"=w967) -> (w966:T8)
              }
              frame "Sample Z Step Size (µm)" {
                n103 = Bundle By Name(cluster=w974, "Z Step Size (µm)"=w973) -> (w972:T8)
              }
            }
            n104 = Bundle By Name(cluster=w932, "Actions"=4Pi_Obj_Lock_-_Actions."Idle") -> (w931:T8)
            n105 = Send Notification(notification=w931, notifier=w934) -> ()  [unwired: 1 in, 2 out]
          }
          event "Sample Z Step No.": Value Change {
            n106 = event-data() -> ("NewVal"=w976:u32)  [unwired: 1 in]
            n107 = for {
              N: w976 -> [_]
              tunnel: [w995] -> w980 mode=indexing
              tunnel: [w984] -> w979 mode=indexing
              i -> [w994]
              w985 = T12 3 items=["Grayscale (U8)", "Grayscale (I16)", "Grayscale (SGL)", "Complex (CSG)", "RGB (U32)", "HSL (U32)", "RGB (U64)", "Grayscale (U16)"] ("Image Type")
              w990 = T12 2 items=["Grayscale (U8)", "Grayscale (I16)", "Grayscale (SGL)", "Complex (CSG)", "RGB (U32)", "HSL (U32)", "RGB (U64)", "Grayscale (U16)"] ("Image Type")
              w986 = 10 ("Border Size")
              n108 = Number To Decimal String(number=w994, width (-)=i16 1) -> (decimal integer string=w992:string)
              n109 = Concatenate Strings("Ref Stack " ("string"), w992) -> (w988:string)
              n110 = call "IMAQ Create"("Border Size"=w986, "Image Name"=w988, "Image Type"=w990) -> ("New Image"=w995:T9)  [unwired: 2 in, 1 out]
              n111 = Concatenate Strings("FFT" ("string"), w988) -> (w987:string)
              n112 = call "IMAQ Create"("Border Size"=w986, "Image Name"=w987, "Image Type"=w985) -> ("New Image"=w984:T9)  [unwired: 2 in, 1 out]
            }
            n113 = Get Notifier Status(notifier=w978) -> (notifier out=w982:refnum<notifier>, current notification=w983:T8)  [unwired: 1 in, 3 out]
            n114 = Bundle By Name(cluster=w983, "Actions"=4Pi_Obj_Lock_-_Actions."Idle", "Z Step No."=w976, "Ref Stack (SGL)"=w980, "Ref FFT Stack (CSG)"=w979) -> (w981:T8)
            n115 = Send Notification(notification=w981, notifier=w982) -> ()  [unwired: 1 in, 2 out]
          }
          event "Frame Accumulations": Value Change {
            n116 = event-data() -> ("NewVal"=w998:u16)  [unwired: 1 in]
            n117 = Get Notifier Status(notifier=w1001) -> (notifier out=w1000:refnum<notifier>, current notification=w999:T8)  [unwired: 1 in, 3 out]
            n118 = Bundle By Name(cluster=w999, "Actions"=4Pi_Obj_Lock_-_Actions."Idle", "Frame Accumulations"=w998) -> (w997:T8)
            n119 = Send Notification(notification=w997, notifier=w1000) -> ()  [unwired: 1 in, 2 out]
          }
          event "Update Delay (ms)": Value Change {
            n120 = event-data() -> ("NewVal"=w1005:i32)  [unwired: 1 in]
            n121 = Get Notifier Status(notifier=w1008) -> (notifier out=w1007:refnum<notifier>, current notification=w1006:T8)  [unwired: 1 in, 3 out]
            n122 = Bundle By Name(cluster=w1006, "Actions"=4Pi_Obj_Lock_-_Actions."Idle", "Update Delay (ms)"=w1005) -> (w1004:T8)
            n123 = Send Notification(notification=w1004, notifier=w1007) -> ()  [unwired: 1 in, 2 out]
          }
          event "Save Lock Settings": Value Change {
            n124 = event-data() -> ()  [unwired: 1 in, 1 out]
            n125 = Wait on Notification(notifier=w1037) -> (notification=w1035:T8)  [unwired: 3 in, 3 out]
            n126 = Unbundle By Name(w1035) -> ("Z Step Size (µm)"=w1011:dbl, "Z Step No."=w1010:u32, "Z Drift Threshold"=w1034:dbl, "Z Stage Move Limit (µm)"=w1033:dbl, "XY Drift Threshold"=w1032:dbl, "XY Stage Move Limit (µm)"=w1031:dbl, "Frame Accumulations"=w1030:u16, "Abort If Error"=w1029:bool, "Z Correction Active"=w1028:bool, "XY Correction Active"=w1027:bool, "PID Values"=w1017:dbl[])
            n127 = local read "Invert X Axis"() -> (w1015:bool)
            n128 = local read "Invert Y Axis"() -> (w1014:bool)
            n129 = local read "Invert Z Axis"() -> (w1013:bool)
            n130 = local read "Flip XY Axis"() -> (w1016:bool)
            n131 = Bundle By Name(cluster=T7 {"Z Drift Threshold"=0.05, "Z Stage Move Limit (µm)"=1.0, "XY Drift Threshold"=0.05, "XY Stage Move Limit (µm)"=1.0, "Frame Accumulations"=10, "Abort If Error"=FALSE, "Flip XY Axis"=FALSE, "Invert X Axis"=FALSE, "Invert Y Axis"=FALSE, "Invert Z Axis"=FALSE, "Z Correction Active"=TRUE, "XY Correction Active"=TRUE, "PID Values"=[], "Update Delay (ms)"=0, "Sample Z Step Size (µm)"=2.0, "Sample Z Step No."=2, "Z Update Scale Factor"=2.0, "Y Update Scale Factor"=2.0, "X Update Scale Factor"=2.0} ("Lock Settings"), "Sample Z Step Size (µm)"=w1011, "Sample Z Step No."=w1010, "Z Drift Threshold"=w1034, "Z Stage Move Limit (µm)"=w1033, "XY Drift Threshold"=w1032, "XY Stage Move Limit (µm)"=w1031, "Frame Accumulations"=w1030, "Abort If Error"=w1029, "Z Correction Active"=w1028, "XY Correction Active"=w1027, "PID Values"=w1017, "Flip XY Axis"=w1016, "Invert X Axis"=w1015, "Invert Y Axis"=w1014, "Invert Z Axis"=w1013) -> (w1026:T7)
            n132 = control-ref of="This VI"() -> (w1024:refnum<vi>)
            n133 = Flatten To JSON(anything=w1026) -> (JSON string=w1019:string)  [unwired: 2 in, 1 out]
            n134 = property class="VI"(reference=w1024) -> ("Path"=w1021:path)  [unwired: 1 in, 2 out]
            n135 = Strip Path(path=w1021) -> (stripped path=w1020:path)  [unwired: 1 out]
            n136 = Build Path(base path=w1020, name or relative path="4Pi Objective Lock Default Settings") -> (appended path=w1022:path)
            n137 = Build Path(base path=w1022, name or relative path="Default Obj Lock Settings.json") -> (appended path=w1018:path)
            n138 = Write to Text File(file (use dialog)=w1018, text=w1019) -> (refnum out=w1012:refnum<file>)  [unwired: 2 in, 2 out]
            n139 = Close File(refnum=w1012) -> ()  [unwired: 1 in, 2 out]
          }
          event "Start Lock": Value Change {
            n140 = event-data() -> ("NewVal"=w1044:bool)  [unwired: 1 in]
            n141 = Select(t=4Pi_Obj_Lock_-_Actions."Start Lock", s=w1044, f=4Pi_Obj_Lock_-_Actions."Abort" ("Actions")) -> (s? t:f=w1042:T6)
            n142 = Get Notifier Status(notifier=w1047) -> (notifier out=w1046:refnum<notifier>, current notification=w1045:T8)  [unwired: 1 in, 3 out]
            n143 = Bundle By Name(cluster=w1045, "Actions"=w1042, "Running?"=TRUE) -> (w1041:T8)
            n144 = Send Notification(notification=w1041, notifier=w1046) -> ()  [unwired: 1 in, 2 out]
          }
          event "Restart Lock": Value Change {
            n145 = event-data() -> ()  [unwired: 1 in, 1 out]
            n146 = Get Notifier Status(notifier=w1054) -> (notifier out=w1053:refnum<notifier>, current notification=w1052:T8)  [unwired: 1 in, 3 out]
            n147 = Bundle By Name(cluster=w1052, "Actions"=4Pi_Obj_Lock_-_Actions."Restart Lock" ("t")) -> (w1051:T8)
            n148 = local write "Start Lock"(TRUE ("Start Lock")) -> ()
            n149 = Send Notification(notification=w1051, notifier=w1053) -> ()  [unwired: 1 in, 2 out]
          }
          event "Quit": Value Change {
            # "Turn off the OBJ lock before quiting."
            n150 = event-data() -> ("NewVal"=w1065:bool)  [unwired: 1 in]
            n151 = Get Notifier Status(notifier=w1060) -> (notifier out=w1058:refnum<notifier>, current notification=w1056:T8)  [unwired: 1 in, 3 out]
            n152 = Unbundle By Name(w1056) -> ("Running?"=w1059:bool)
            n153 = case shown="True" w1059 {
              tunnel: w1058 -> [w1066 w1070]
              tunnel: [w1066 w1067] -> w1057
              tunnel: w1056 -> [_ w1072]
              frame False {
              }
              frame True {
                n154 = Bundle By Name(cluster=w1072, "Actions"=4Pi_Obj_Lock_-_Actions."Abort") -> (w1069:T8)
                n155 = Send Notification(notification=w1069, notifier=w1070) -> (notifier out=w1068:refnum<notifier>)  [unwired: 1 in, 1 out]
                n156 = while {
                  tunnel: w1068 -> [w1082]
                  tunnel: [w1077] -> w1067
                  i -> [w1076]
                  stop <- w1078 stop-if-true
                  n157 = Get Notifier Status(notifier=w1082) -> (notifier out=w1077:refnum<notifier>, # waiting=w1081:i32)  [unwired: 1 in, 3 out]
                  n158 = Greater?(x=w1076, y=1500) -> (0:w1074:bool)
                  n159 = Less?(x=w1081, y=1) -> (x < y?=w1079:bool)
                  n160 = Or(x=w1079, y=w1074) -> (x .or. y?=w1078:bool)
                  n161 = Wait (ms)(milliseconds to wait=u32 1) -> ()  [unwired: 1 out]
                }
              }
            }
            n162 = Get Notifier Status(notifier=w1057) -> (notifier out=w1062:refnum<notifier>, current notification=w1064:T8)  [unwired: 1 in, 3 out]
            n163 = Bundle By Name(cluster=w1064, "Actions"=4Pi_Obj_Lock_-_Actions."Quit") -> (w1061:T8)
            n164 = Send Notification(notification=w1061, notifier=w1062) -> ()  [unwired: 1 in, 2 out]
          }
        }
      }
      n165 = while {
        tunnel: w193 -> [w219]
        tunnel: w191 -> [w207]
        tunnel: w190 -> [w206]
        tunnel: w192 -> [w218]
        stop <- w214 stop-if-true
        # "Column 1 - Target Lock Values\nColumn 2 - Current Values\nColumn 3 - Differnce Values\nColumn 4 - Initial XYZ Stage Positions"
        n166 = Wait on Notification(notifier=w218, ignore previous (F)=FALSE) -> (notifier out=w213:refnum<notifier>, notification=w216:T8)  [unwired: 2 in, 2 out]
        n167 = Unbundle By Name(w216) -> ("Actions"=w208:T6)
        n168 = Equal?(x=4Pi_Obj_Lock_-_Actions."Quit", y=w208) -> (x = y?=w214:bool)
        n169 = Initialize Array(0.0 ("element"), 3 ("dimension size"), 4 ("dimension size")) -> (w210:dbl[][])
        n170 = while {
          shift-right: [w226] -> _
          shift-left: w208 -> [w234]
          tunnel: w219 -> [w238]
          tunnel: w207 -> [w237]
          tunnel: w206 -> [w236]
          tunnel: w213 -> [w232]
          shift-right: [w220] -> _
          shift-left: w210 -> [w221]
          stop <- w233 stop-if-true
          w228 = 4Pi_Obj_Lock_-_Actions."Abort" ("x")
          n171 = case shown="\"Start Lock\"" w234 {
            selector: w234 -> [_ _ _ _ _ _ _ _ _ _ _ w695 _ _ _ _ _ _]
            tunnel: w238 -> [_ w270 _ w341 _ w404 w476 w510 w548 w583 _ _ _ _ _ w864 _ _]
            tunnel: w237 -> [_ w279 _ _ _ _ w452 _ _ _ _ w699 _ _ _ _ _ _]
            tunnel: w236 -> [_ w278 w299 w342 _ w419 w451 _ _ _ _ _ w770 _ _ _ _ _]
            tunnel: FALSE -> [w241 w291 w295 w340 w391 w415 w479 w541 w550 w613 w665 w730 w775 w842 w851 w868 _ _]
            tunnel: [4Pi_Obj_Lock_-_Actions."Exit Loop" ("x") 4Pi_Obj_Lock_-_Actions."Get Target Z Position" ("x") 4Pi_Obj_Lock_-_Actions."Get Ref Stack" ("x") w345 4Pi_Obj_Lock_-_Actions."Move To Init Z" ("x") w400 w471 w524 w553 w600 w643 w714 w751 4Pi_Obj_Lock_-_Actions."Delay" ("x") 4Pi_Obj_Lock_-_Actions."Get Current Z Position" ("x") 4Pi_Obj_Lock_-_Actions."Exit Loop" ("x") 4Pi_Obj_Lock_-_Actions."Exit Loop" ("x") 4Pi_Obj_Lock_-_Actions."Quit" ("x")] -> w227
            tunnel: [w241 w291 w295 w340 w391 w415 w479 w541 w550 w613 w665 w730 w775 w842 w851 w868 TRUE TRUE] -> w233
            tunnel: w232 -> [w240 w259 w300 w344 w396 w413 w478 w540 w563 w612 w664 w729 w773 w840 w849 w872 w878 w882]
            tunnel: [w240 w252 w298 w343 w393 w413 w478 w532 w562 w611 w663 w728 w772 w839 w845 w871 w878 w881] -> w231
            tunnel: w221 -> [w239 w275 w294 w339 w390 w414 w464 w539 w549 w588 w653 w685 w749 w820 w848 w867 w877 w890]
            tunnel: [w239 w274 w294 w339 w390 w414 w463 w538 w549 w587 w650 w685 w749 w820 w848 w867 w877 w890] -> w220
            frame "Idle", Default {
            }
            frame "Start Lock" {
              w251 = T17 [] ("History Data")
              w271 = FALSE ("Move Limit Error")
              w276 = Stage_Actions."Get Position" ("Actions")
              n172 = control-ref of="This VI"() -> (w289:refnum<vi>)
              n173 = call "Stages Messenger.vi"("Stage Notifier Name"=w279, "Actions"=w276) -> ("Positions"=w280:dbl[])  [unwired: 10 in, 3 out]
              n174 = call "Stages Messenger.vi"("Stage Notifier Name"=w278, "Actions"=w276) -> ("Positions"=w281:dbl[])  [unwired: 10 in, 3 out]
              n175 = property class="VI"(reference=w289) -> ("Path"=w286:path)  [unwired: 1 in, 2 out]
              n176 = local write "Move Limit Error"(w271) -> ()
              n177 = local write "Fit Error"(w271) -> ()
              n178 = Index Array(array=w281, index=0) -> (element=w277:dbl)
              n179 = Strip Path(path=w286) -> (stripped path=w285:path)  [unwired: 1 out]
              n180 = Build Path(base path=w285, name or relative path="4Pi Objective Lock Default Settings") -> (appended path=w287:path)
              n181 = Build Array (concatenate)(w280, w277) -> (w249:dbl[])
              n182 = Build Path(base path=w287, name or relative path="Initial Stage Positions.json") -> (appended path=w283:path)
              n183 = Flatten To JSON(anything=w249) -> (JSON string=w284:string)  [unwired: 2 in, 1 out]
              n184 = Replace Array Subset(array=w275, new element=w249, index (col)=3 ("disabled index (col)")) -> (w274:dbl[][])  [unwired: 1 in]
              n185 = Index Array(array=w249, index #1=0 ("index"), index #2=1 ("index"), index #3=2 ("index")) -> (element #1=w245:dbl, element #2=w243:dbl, element #3=w244:dbl)
              n186 = Write to Text File(file (use dialog)=w283, text=w284) -> (refnum out=w272:refnum<file>)  [unwired: 2 in, 2 out]
              n187 = local write "X Axis Position (µm)"(w245) -> ()
              n188 = local write "Y Axis Position (µm)"(w243) -> ()
              n189 = local write "Z Axis Position (µm)"(w244) -> ()
              n190 = Get Notifier Status(notifier=w259) -> (notifier out=w252:refnum<notifier>, current notification=w257:T8)  [unwired: 1 in, 3 out]
              n191 = Close File(refnum=w272) -> ()  [unwired: 1 in, 2 out]
              n192 = Unbundle By Name(w257) -> ("Cur Image (SGL)"=w256:T9)
              n193 = Unbundle By Name(w257) -> ("Z Step No."=w254:u32, "Ref Stack (SGL)"=w253:T9[])
              n194 = call "Camera Messenger.vi"("Notifier Name"=w270, "General Camera Actions"=Generic_Camera_Actions."Record Settings", "No. of Frames"=u32 1) -> ("Notifier Name Dup"=w268:string)  [unwired: 7 in, 5 out]
              n195 = call "Camera Messenger.vi"("Notifier Name"=w268, "General Camera Actions"=Generic_Camera_Actions."Get ROI", "Camera ROI"=T14 {"H_Offset"=0, "V_Offset"=0, "H_Width"=0, "V_Width"=0} ("General Camera ROI")) -> ("Camera ROI"=w260:T14)  [unwired: 7 in, 5 out]
              n196 = Unbundle By Name(w260) -> ("H_Width"=w265:u16, "V_Width"=w263:u16)
              n197 = To Long Integer(number=w265) -> (32bit integer=w264:i32)
              n198 = To Long Integer(number=w263) -> (32bit integer=w262:i32)
              n199 = Initialize Array(sgl 0.0 ("element"), w264, w262) -> (w255:sgl[][])
              n200 = for {
                N: w254 -> [_]
                tunnel: w255 -> [w292]
                tunnel: w253 -> [w293] mode=indexing
                n201 = call "IMAQ ArrayToImage"("Image Pixels (Float)"=w292, "Image"=w293) -> ()  [unwired: 8 in, 2 out]
              }
              n202 = call "IMAQ ArrayToImage"("Image Pixels (Float)"=w255, "Image"=w256) -> ()  [unwired: 8 in, 2 out]
              n203 = property on="X Target and Fit Position (µm)" class="WFChart (strict)"("History Data"=w251) -> ()  [unwired: 2 in, 2 out]
              n204 = property on="Y Target and Fit Position (µm)" class="WFChart (strict)"("History Data"=w251) -> ()  [unwired: 2 in, 2 out]
              n205 = property on="Z Target and Fit Value (µm)" class="WFChart (strict)"("History Data"=w251) -> ()  [unwired: 2 in, 2 out]
            }
            frame "Get Target Z Position" {
              w322 = 0.0 ("Target Z (µm)")
              n206 = Get Notifier Status(notifier=w300) -> (notifier out=w320:refnum<notifier>, current notification=w325:T8)  [unwired: 1 in, 3 out]
              n207 = Unbundle By Name(w325) -> ("Z Step No."=w318:u32, "Z Step Size (µm)"=w317:dbl, "Z Stage Move Limit (µm)"=w315:dbl)
              n208 = Unbundle By Name(w325) -> ("Z Step No."=w310:u32, "Z Step Size (µm)"=w323:dbl)
              n209 = Divide(x=w318, y=2.0) -> (x/y=w308:dbl)
              n210 = Round Toward -Infinity(1:w308) -> (0:w307:dbl)
              n211 = Multiply(x=w307, y=w317) -> (x*y=w312:dbl)
              n212 = Decrement(x=w310) -> (x-1=w309:u32)
              n213 = Negate(x=w312) -> (-x=w311:dbl)
              n214 = Negate(x=w315) -> (-x=w316:dbl)
              n215 = In Range and Coerce(upper limit=w315, x=w311, lower limit=w316) -> (coerced(x)=w313:dbl)  [unwired: 1 out]
              n216 = Add(x=w322, y=w313) -> (x+y=w314:dbl)
              n217 = Build Array(w314) -> (w324:dbl[])
              n218 = for {
                N: w309 -> [_]
                tunnel: w323 -> [w336]
                shift-right: [w337] -> w321
                shift-left: w324 -> [w338]
                shift-right: [w334] -> _
                shift-left: w314 -> [w335]
                n219 = Add(x=w335, y=w336) -> (x+y=w334:dbl)
                n220 = Build Array (concatenate)(w338, w334) -> (w337:dbl[])
              }
              n221 = Build Array(w313) -> (w326:dbl[])
              n222 = call "Stages Messenger.vi"("Stage Notifier Name"=w299, "Actions"=Stage_Actions."MVR", "Setpoint"=w326, "Axis"=bool[] [TRUE], "Exit While Busy?"=TRUE) -> ("Stage Notifier Name (Dup)"=w305:string, "Status"=w306:T18)  [unwired: 7 in, 2 out]
              n223 = case shown="Default" w306 {
                tunnel: [w332] -> w304
                tunnel: w305 -> [w332]
                frame Default {
                  n224 = Wait (ms)(milliseconds to wait=u32 250) -> ()  [unwired: 1 out]
                }
              }
              n225 = Bundle By Name(cluster=w325, "Sample Z (µm)"=w321) -> (w319:T8)
              n226 = call "Stages Messenger.vi"("Stage Notifier Name"=w304, "Actions"=Stage_Actions."Get Position", "Exit While Busy?"=TRUE) -> ("Positions"=w302:dbl[])  [unwired: 9 in, 3 out]
              n227 = Index Array(array=w302, index=0) -> (element=w296:dbl)
              n228 = Send Notification(notification=w319, notifier=w320) -> (notifier out=w298:refnum<notifier>)  [unwired: 1 in, 1 out]
              n229 = local write "Z Axis Position (µm)"(w296) -> ()
              "Target Z (µm)" <- w322
            }
            frame "Get Ref Stack" {
              n230 = Get Notifier Status(notifier=w344) -> (notifier out=w343:refnum<notifier>, current notification=w349:T8)  [unwired: 1 in, 3 out]
              n231 = Unbundle By Name(w349) -> ("Z Step No."=w348:u32, "Ref Stack (SGL)"=w347:T9[])
              n232 = Unbundle By Name(w349) -> ("Z Step Size (µm)"=w346:dbl)
              n233 = while {
                tunnel: w341 -> [w366]
                tunnel: w348 -> [w363]
                tunnel: w343 -> [w365]
                tunnel: [w355] -> w345
                tunnel: w347 -> [w354] mode=indexing
                tunnel: w346 -> [w353]
                tunnel: w342 -> [w352]
                i -> [w362]
                stop <- w358 stop-if-true
                n234 = flat-sequence {
                  tunnel: w366 -> [w372]
                  tunnel: w354 -> [w369]
                  tunnel: w353 -> [w384]
                  tunnel: w352 -> [w383]
                  frame #0 {
                    w370 = T12 2 items=["Grayscale (U8)", "Grayscale (I16)", "Grayscale (SGL)", "Complex (CSG)", "RGB (U32)", "HSL (U32)", "RGB (U64)", "Grayscale (U16)"] ("Image Type")
                    n235 = call "Camera Messenger.vi"("Notifier Name"=w372, "General Camera Actions"=Generic_Camera_Actions."Capture") -> ("Notifier Name Dup"=w368:string)  [unwired: 8 in, 5 out]
                    n236 = while {
                      tunnel: w368 -> [w382]
                      tunnel: [w375] -> w367
                      i -> [w378]
                      stop <- w376 stop-if-true
                      n237 = call "Camera Messenger.vi"("Notifier Name"=w382, "General Camera Actions"=Generic_Camera_Actions."Status") -> ("Running?"=w374:bool, "Image Ref"=w375:T9)  [unwired: 8 in, 4 out]
                      n238 = Not(x=w374) -> (.not. x?=w373:bool)
                      n239 = Greater?(x=w378, y=500) -> (0:w380:bool)
                      n240 = Wait (ms)(milliseconds to wait=u32 1) -> ()  [unwired: 1 out]
                      n241 = Or(x=w373, y=w380) -> (x .or. y?=w376:bool)
                    }
                    n242 = call "IMAQ Cast Image"("Image Type"=w370, "Image Dst"=w369, "Image Src"=w367) -> ()  [unwired: 7 in, 2 out]
                  }
                  frame #1 {
                    n243 = Build Array(w384) -> (w388:dbl[])
                    n244 = Wait (ms)(milliseconds to wait=u32 250) -> ()  [unwired: 1 out]
                    n245 = call "Stages Messenger.vi"("Stage Notifier Name"=w383, "Actions"=Stage_Actions."MVR", "Setpoint"=w388, "Axis"=bool[] [TRUE], "Exit While Busy?"=TRUE) -> ()  [unwired: 7 in, 4 out]
                  }
                }
                n246 = Get Notifier Status(notifier=w365) -> (current notification=w357:T8)  [unwired: 1 in, 4 out]
                n247 = To Unsigned Long Integer(number=w362) -> (unsigned 32bit integer=w361:u32)
                n248 = Increment(x=w361) -> (x+1=w364:u32)
                n249 = Unbundle By Name(w357) -> ("Running?"=w360:bool)
                n250 = Greater Or Equal?(x=w364, y=w363) -> (x >= y?=w359:bool)
                n251 = Not(x=w360) -> (.not. x?=w356:bool)
                n252 = Or(x=w356, y=w359) -> (x .or. y?=w358:bool)
                n253 = Select(t=4Pi_Obj_Lock_-_Actions."Abort" ("x"), s=w356, f=4Pi_Obj_Lock_-_Actions."Cal Ref FFT") -> (s? t:f=w355:T6)
              }
            }
            frame "Cal Ref FFT" {
              n254 = Get Notifier Status(notifier=w396) -> (notifier out=w393:refnum<notifier>, current notification=w397:T8)  [unwired: 1 in, 3 out]
              n255 = Unbundle By Name(w397) -> ("Ref Stack (SGL)"=w395:T9[], "Ref FFT Stack (CSG)"=w394:T9[])
              n256 = for {
                tunnel: w395 -> [w399] mode=indexing
                tunnel: w394 -> [w398] mode=indexing
                n257 = call "4Pi Obj Lock - Norm FFT.vi"("FFT Image Dst"=w398, "Image In"=w399) -> ()  [unwired: 8 in, 2 out]
              }
            }
            frame "Move To Init Z" {
              # "initial z stage position"
              n258 = call "Camera Messenger.vi"("Notifier Name"=w404, "General Camera Actions"=Generic_Camera_Actions."Live Preview") -> ("Notifier Name Dup"=w406:string)  [unwired: 8 in, 5 out]
              n259 = Index Array(array=w414, index (row)=2, index (col)=3 ("disabled index (col)")) -> (element=w416:dbl)
              n260 = while {
                tunnel: w406 -> [w428]
                tunnel: [w423] -> w403
                i -> [w427]
                stop <- w424 stop-if-true
                n261 = call "Camera Messenger.vi"("Notifier Name"=w428, "General Camera Actions"=Generic_Camera_Actions."Status") -> ("Running?"=w425:bool)  [unwired: 8 in, 5 out]
                n262 = Greater?(x=w427, y=3000) -> (0:w423:bool)
                n263 = Or(x=w425, y=w423) -> (x .or. y?=w424:bool)
                n264 = Wait (ms)(milliseconds to wait=u32 1) -> ()  [unwired: 1 out]
              }
              n265 = flat-sequence {
                tunnel: w419 -> [w437]
                tunnel: [w436] -> w421
                tunnel: w416 -> [w432]
                tunnel: [w430] -> w420
                tunnel: w421 -> [w442]
                tunnel: w420 -> [w441]
                tunnel: [w440] -> w407
                frame #0 {
                  n266 = call "Stages Messenger.vi"("Stage Notifier Name"=w437, "Actions"=Stage_Actions."Get Position") -> ("Stage Notifier Name (Dup)"=w436:string, "Positions"=w434:dbl[])  [unwired: 10 in, 2 out]
                  n267 = Index Array(array=w434, index=0) -> (element=w433:dbl)
                  n268 = Subtract(x=w432, y=w433) -> (x-y=w431:dbl)
                  n269 = Build Array(w431) -> (w430:dbl[])
                }
                frame #1 {
                  n270 = Wait (ms)(milliseconds to wait=u32 250) -> ()  [unwired: 1 out]
                  n271 = call "Stages Messenger.vi"("Stage Notifier Name"=w442, "Actions"=Stage_Actions."MVR", "Setpoint"=w441, "Axis"=bool[] [TRUE], "Exit While Busy?"=TRUE) -> ("Stage Notifier Name (Dup)"=w440:string)  [unwired: 7 in, 3 out]
                }
              }
              n272 = call "Stages Messenger.vi"("Stage Notifier Name"=w407, "Actions"=Stage_Actions."Get Position", "Exit While Busy?"=TRUE) -> ("Positions"=w410:dbl[])  [unwired: 9 in, 3 out]
              n273 = Index Array(array=w410, index=0) -> (element=w408:dbl)
              n274 = local write "Z Axis Position (µm)"(w408) -> ()
              n275 = Select(t=4Pi_Obj_Lock_-_Actions."Exit Loop", s=w403, f=4Pi_Obj_Lock_-_Actions."Get Initial Position" ("x")) -> (s? t:f=w400:T6)
            }
            frame "Restart Lock" {
              w446 = T17 [] ("History Data")
              w447 = FALSE ("Move Limit Error")
              # "Make sure the camera is running, if not abort."
              n276 = control-ref of="This VI"() -> (w469:refnum<vi>)
              n277 = call "Camera Messenger.vi"("Notifier Name"=w476, "General Camera Actions"=Generic_Camera_Actions."Live Preview") -> ("Notifier Name Dup"=w475:string)  [unwired: 8 in, 5 out]
              n278 = property class="VI"(reference=w469) -> (error out=w455:errorcluster, "Path"=w466:path)  [unwired: 1 in, 1 out]
              n279 = while {
                tunnel: w475 -> [w505]
                tunnel: [w500] -> w474
                i -> [w504]
                stop <- w501 stop-if-true
                n280 = call "Camera Messenger.vi"("Notifier Name"=w505, "General Camera Actions"=Generic_Camera_Actions."Status") -> ("Running?"=w502:bool)  [unwired: 8 in, 5 out]
                n281 = Greater?(x=w504, y=3000) -> (0:w500:bool)
                n282 = Or(x=w502, y=w500) -> (x .or. y?=w501:bool)
                n283 = Wait (ms)(milliseconds to wait=u32 1) -> ()  [unwired: 1 out]
              }
              n284 = Strip Path(path=w466) -> (stripped path=w465:path)  [unwired: 1 out]
              n285 = Build Path(base path=w465, name or relative path="4Pi Objective Lock Default Settings") -> (appended path=w467:path)
              n286 = Build Path(base path=w467, name or relative path="Initial Stage Positions.json") -> (appended path=w461:path)
              n287 = Read from Text File(file (use dialog)=w461, error in=w455) -> (refnum out=w460:refnum<file>, text=w459:string, error out=w458:errorcluster)  [unwired: 2 in, 1 out]
              n288 = Close File(refnum=w460, error in=w458) -> (error out=w457:errorcluster)  [unwired: 1 out]
              n289 = local write "Move Limit Error"(w447) -> ()
              n290 = local write "Fit Error"(w447) -> ()
              n291 = Unflatten From JSON(JSON string=w459, type and defaults=dbl[] [], error in (no error)=w457) -> (value=w453:dbl[], error out=w454:errorcluster)  [unwired: 4 in]
              n292 = case shown="Error" w454 {
                tunnel: w453 -> [w481 _]
                tunnel: w452 -> [w488 w493]
                tunnel: w451 -> [w487 w492]
                tunnel: [w481 w491] -> w450
                tunnel: u32 150 ("milliseconds to wait") -> [w480 w490]
                tunnel: [w480 w490] -> w448
                frame No Error {
                  w489 = Stage_Actions."MOVE" ("Actions")
                  n293 = Split 1D Array(array=w481, index=2) -> (first subarray=w485:dbl[], second subarray=w484:dbl[])
                  n294 = call "Stages Messenger.vi"("Stage Notifier Name"=w488, "Actions"=w489, "Setpoint"=w485, "Axis"=bool[] [TRUE, TRUE]) -> ()  [unwired: 8 in, 4 out]
                  n295 = call "Stages Messenger.vi"("Stage Notifier Name"=w487, "Actions"=w489, "Setpoint"=w484, "Axis"=bool[] [TRUE]) -> ()  [unwired: 8 in, 4 out]
                }
                frame Error {
                  w494 = Stage_Actions."Get Position" ("Actions")
                  n296 = call "Stages Messenger.vi"("Stage Notifier Name"=w493, "Actions"=w494) -> ("Positions"=w496:dbl[])  [unwired: 10 in, 3 out]
                  n297 = call "Stages Messenger.vi"("Stage Notifier Name"=w492, "Actions"=w494) -> ("Positions"=w497:dbl[])  [unwired: 10 in, 3 out]
                  n298 = Index Array(array=w497, index=0) -> (element=w495:dbl)
                  n299 = Build Array (concatenate)(w496, w495) -> (w491:dbl[])
                }
              }
              n300 = Wait (ms)(milliseconds to wait=w448) -> ()  [unwired: 1 out]
              n301 = property on="X Target and Fit Position (µm)" class="WFChart (strict)"("History Data"=w446) -> ()  [unwired: 2 in, 2 out]
              n302 = property on="Y Target and Fit Position (µm)" class="WFChart (strict)"("History Data"=w446) -> ()  [unwired: 2 in, 2 out]
              n303 = property on="Z Target and Fit Value (µm)" class="WFChart (strict)"("History Data"=w446) -> ()  [unwired: 2 in, 2 out]
              n304 = Replace Array Subset(array=w464, new element=w450, index (col)=3 ("disabled index (col)")) -> (w463:dbl[][])  [unwired: 1 in]
              n305 = Select(t=4Pi_Obj_Lock_-_Actions."Exit Loop" ("x"), s=w474, f=4Pi_Obj_Lock_-_Actions."Get Initial Position" ("x")) -> (s? t:f=w471:T6)
            }
            frame "Get Initial Position" {
              w517 = 0 ("index")
              # "Set target values"
              n306 = Get Notifier Status(notifier=w540) -> (notifier out=w533:refnum<notifier>, current notification=w508:T8)  [unwired: 1 in, 3 out]
              n307 = Unbundle By Name(w508) -> ("Frame Accumulations"=w507:u16)
              n308 = Bundle By Name(cluster=w508, "Running?"=TRUE) -> (w530:T8)
              n309 = Send Notification(notification=w530, notifier=w533) -> (notifier out=w532:refnum<notifier>)  [unwired: 1 in, 1 out]
              n310 = call "Generic Camera Get New Camera Image.vi"("Camera Notifier Name"=w510, "Frames"=w507) -> ("Image - U16"=w509:u16[][])  [unwired: 11 in, 2 out]
              n311 = call "2D Gaussian - Fit Image U16.vi"("Image In (U16)"=w509) -> ("Best Fit Params"=w537:T19, "Error Out"=w523:errorcluster)  [unwired: 13 in]
              n312 = Unbundle By Name(w523) -> ("status"=w522:bool)
              n313 = Cluster To Array(cluster=w537) -> (array=w536:dbl[])
              n314 = local write "Fit Error"(w522) -> ()
              n315 = Array Subset(array=w536, index=1, length=4) -> (w529:dbl[])
              n316 = Index Array(array=w529, index #1=0 ("index"), index #2=1 ("index"), index #3=2 ("index"), index #4=3 ("index")) -> (element #1=w511:dbl, element #2=w512:dbl, element #3=w519:dbl, element #4=w518:dbl)
              "Target X Position (px)" <- w511
              "Target Y Position (px)" <- w512
              n317 = Divide(x=w519, y=w518) -> (x/y=w513:dbl)
              "Target sx/sy" <- w513
              n318 = Replace Array Subset(array=w539, new element #1=w511, index (row) #1=0 ("disabled index (row)"), index (col) #1=w517, new element #2=w512, index (row) #2=1 ("disabled index (row)"), index (col) #2=w517, new element #3=w513, index (row) #3=2 ("disabled index (row)"), index (col) #3=w517) -> (w538:dbl[][])
              n319 = Select(t=4Pi_Obj_Lock_-_Actions."Abort" ("x"), s=w522, f=4Pi_Obj_Lock_-_Actions."Get Current Z Position" ("x")) -> (s? t:f=w524:T6)
            }
            frame "Get Current Z Position" {
              n320 = Get Notifier Status(notifier=w563) -> (notifier out=w562:refnum<notifier>, current notification=w547:T8)  [unwired: 1 in, 3 out]
              n321 = Unbundle By Name(w547) -> ("CC Image (SGL)"=w554:T9)
              n322 = Unbundle By Name(w547) -> ("Ref FFT Stack (CSG)"=w569:T9[])
              n323 = Unbundle By Name(w547) -> ("Cur Image (SGL)"=w543:T9, "Tmp Image FFT (CSG)"=w559:T9[])
              n324 = Unbundle By Name(w547) -> ("Sample Z (µm)"=w571:dbl[])
              n325 = Unbundle By Name(w547) -> ("Frame Accumulations"=w546:u16)
              n326 = call "Generic Camera Get New Camera Image.vi"("Camera Notifier Name"=w548, "Frames"=w546) -> ("Image - U16"=w545:u16[][])  [unwired: 11 in, 2 out]
              n327 = Index Array(array=w559, index #1=0 ("index"), index #2=1 ("index"), index #3=2 ("index")) -> (element #1=w557:T9, element #2=w555:T9, element #3=w556:T9)
              n328 = To Single Precision Float(number=w545) -> (single precision float=w542:sgl[][])
              n329 = call "IMAQ ArrayToImage"("Image Pixels (Float)"=w542, "Image"=w543) -> ("Image Out"=w544:T9)  [unwired: 8 in, 1 out]
              n330 = call "4Pi Obj Lock - Norm FFT.vi"("FFT Image Dst"=w557, "Image In"=w544) -> ("FFT Image Out"=w567:T9)  [unwired: 8 in, 1 out]
              n331 = call "IMAQ ComplexConjugate"("Image Src"=w567) -> ("Image Dst Out"=w566:T9)  [unwired: 3 in, 1 out]
              n332 = for {
                tunnel: w554 -> [w578]
                tunnel: [w577] -> w572 mode=indexing
                tunnel: w566 -> [w576]
                tunnel: w569 -> [w575] mode=indexing
                tunnel: w556 -> [w574]
                tunnel: w555 -> [w573]
                n333 = call "4Pi Obj Lock - Get Cross Correlation.vi"("Ref FFT image"=w575, "Cur FFT Image"=w576, "FFT CC image"=w573, "iFFT image"=w574, "CC image"=w578) -> ("Max CC"=w577:sgl)  [unwired: 9 in, 1 out]
              }
              n334 = To Double Precision Float(number=w572) -> (double precision float=w568:dbl[])
              n335 = call "4Pi Obj Lock - Find Peak Position.vi"("Fit Size"=2, "y"=w568, "x"=w571) -> ("Coerced Peak Position"=w565:dbl)  [unwired: 7 in, 1 out]
              "Measured Z (µm)" <- w565
              n336 = Not A Number/Path/Refnum?(number/path/refnum=w565) -> (NaN/Path/Refnum?=w564:bool)
              n337 = Select(t=4Pi_Obj_Lock_-_Actions."Get Current Z Position" ("x"), s=w564, f=4Pi_Obj_Lock_-_Actions."Get Current Position") -> (s? t:f=w553:T6)
            }
            frame "Get Current Position" {
              w592 = 1 ("index")
              # "retake current image"
              # "Update current values"
              n338 = Get Notifier Status(notifier=w612) -> (notifier out=w611:refnum<notifier>, current notification=w580:T8)  [unwired: 1 in, 3 out]
              n339 = Unbundle By Name(w580) -> ("Abort If Error"=w605:bool, "Cur Image (SGL)"=w582:T9)
              n340 = case shown="True" FALSE {
                tunnel: w583 -> [_ w622]
                tunnel: w582 -> [w616 w619]
                tunnel: w580 -> [_ w621]
                tunnel: [w614 w618] -> w579
                frame False {
                  n341 = call "IMAQ ImageToArray"("Image"=w616) -> ("Image Pixels (Float)"=w615:sgl[][])  [unwired: 3 in, 4 out]
                  n342 = To Unsigned Word Integer(number=w615) -> (unsigned 16bit integer=w614:u16[][])
                }
                frame True {
                  n343 = Unbundle By Name(w621) -> ("Frame Accumulations"=w620:u16)
                  n344 = call "Generic Camera Get New Camera Image.vi"("Camera Notifier Name"=w622, "Frames"=w620) -> ("Image - U16"=w618:u16[][])  [unwired: 11 in, 2 out]
                  n345 = To Single Precision Float(number=w618) -> (single precision float=w617:sgl[][])
                  n346 = call "IMAQ ArrayToImage"("Image Pixels (Float)"=w617, "Image"=w619) -> ()  [unwired: 8 in, 2 out]
                }
              }
              n347 = call "2D Gaussian - Fit Image U16.vi"("Image In (U16)"=w579) -> ("Best Fit Params"=w610:T19, "Error Out"=w606:errorcluster)  [unwired: 13 in]
              n348 = Unbundle By Name(w606) -> ("status"=w604:bool)
              "Fit Error" <- w604
              n349 = And(x=w605, y=w604) -> (x .and. y?=w603:bool)
              n350 = Cluster To Array(cluster=w610) -> (array=w609:dbl[])
              n351 = Array Subset(array=w609, index=1, length=4) -> (w593:dbl[])
              n352 = Index Array(array=w593, index #1=0 ("index"), index #2=1 ("index"), index #3=2 ("index"), index #4=3 ("index")) -> (element #1=w584:dbl, element #2=w585:dbl, element #3=w595:dbl, element #4=w594:dbl)
              "Measured X Position (px)" <- w584
              "Measured Y Position (px)" <- w585
              n353 = Divide(x=w595, y=w594) -> (x/y=w586:dbl)
              "Measured sx/sy" <- w586
              n354 = Select(t=4Pi_Obj_Lock_-_Actions."Abort" ("x"), s=w603, f=4Pi_Obj_Lock_-_Actions."Check Drift" ("x")) -> (s? t:f=w600:T6)
              n355 = Replace Array Subset(array=w588, new element #1=w584, index (row) #1=0 ("disabled index (row)"), index (col) #1=w592, new element #2=w585, index (row) #2=1 ("disabled index (row)"), index (col) #2=w592, new element #3=w586, index (row) #3=2 ("disabled index (row)"), index (col) #3=w592) -> (w587:dbl[][])
            }
            frame "Check Drift" {
              # "Update the PID difference between target values and current values"
              # "Check if Sigma X / Sigma Y is over the limit"
              # "Check if XY values are over the limit"
              n356 = Get Notifier Status(notifier=w664) -> (notifier out=w663:refnum<notifier>, current notification=w662:T8)  [unwired: 1 in, 3 out]
              n357 = Unbundle By Name(w662) -> ("Z Correction Active"=w639:bool, "XY Correction Active"=w641:bool, "XY Drift Threshold"=w624:dbl, "Z Drift Threshold"=w632:dbl, "PID Values"=w661:dbl[])
              n358 = local read "Measured Z (µm)"() -> (w633:dbl)
              n359 = local read "Target Z (µm)"() -> (w635:dbl)
              n360 = Index Array(array=w653, index (col) #1=0 ("disabled index (col)"), index (col) #2=1 ("index (col)")) -> (element #1=w655:dbl[], element #2=w654:dbl[])  [unwired: 2 in]
              n361 = Array To Cluster(array=w661) -> (cluster=w634:T20)
              n362 = local read "pixel size (µm)"() -> (w623:dbl)
              n363 = Build Array(w634) -> (w660:T21)
              n364 = Divide(x=w624, y=w623) -> (x/y=w625:dbl)
              n365 = call-poly <vilib>:"PID.vi"("PID gains"=w634, "process variable"=w633, "setpoint"=w635) -> ("output"=w626:dbl)  [unwired: 7 in, 1 out]
              "dz (µm)" <- w626
              n366 = call-poly <vilib>:"PID.vi"("PID gains"=w660, "process variable"=w654, "setpoint"=w655) -> ("output"=w651:dbl[])  [unwired: 7 in, 1 out]
              n367 = Build Array(w625, w625, w632) -> (w658:dbl[])
              n368 = Replace Array Subset(array=w653, new element=w651, index (col)=2 ("disabled index (col)")) -> (w650:dbl[][])  [unwired: 1 in]
              n369 = Absolute Value(x=w651) -> (abs(x)=w659:dbl[])
              n370 = Absolute Value(x=w626) -> (abs(x)=w631:dbl)
              n371 = Greater?(x=w659, y=w658) -> (0:w649:bool[])
              n372 = Greater?(x=w631, y=w632) -> (0:w630:bool)
              n373 = Split 1D Array(array=w649, index=2) -> (first subarray=w647:bool[], second subarray=w646:bool[])
              n374 = Or Array Elements(Boolean array=w647) -> (logical OR=w642:bool)
              n375 = Or Array Elements(Boolean array=w646) -> (logical OR=w629:bool)
              n376 = Select(t=w629, s=FALSE, f=w630) -> (s? t:f=w627:bool)
              n377 = And(x=w641, y=w642) -> (x .and. y?=w640:bool)
              n378 = And(x=w639, y=w627) -> (x .and. y?=w638:bool)
              n379 = Build Array(w640, w638) -> (w645:bool[])
              n380 = Boolean Array To Number(Boolean array=w645) -> (number=w644:u32)
              n381 = case shown="0, Default" w644 {
                tunnel: [4Pi_Obj_Lock_-_Actions."Update Plots" ("x") 4Pi_Obj_Lock_-_Actions."Move XY" ("x") 4Pi_Obj_Lock_-_Actions."Move Z" ("x") 4Pi_Obj_Lock_-_Actions."Move XYZ" ("x")] -> w643
                tunnel: [w666 TRUE FALSE w674] -> w637
                tunnel: [w666 FALSE TRUE w674] -> w636
                frame 0, Default {
                  w666 = FALSE
                  # "XYZ within limits, no move"
                }
                frame 1 {
                  # "X or Y outside limit, move XY"
                }
                frame 2 {
                  # "Sigma X / Y outside limit, move Z"
                }
                frame 3 {
                  w674 = TRUE
                  # "XYZ outside limit, move all"
                }
              }
              "XY Move" <- w637
              "Z Move" <- w636
            }
            frame "Move XYZ", "Move XY" {
              w707 = 2.0
              # "Initial XY stage positions"
              # "Column 3"
              # "Row 1"
              # "Check if move will go beyond ±2 µm of the original positions"
              # "Get XY Diff Values"
              n382 = Get Notifier Status(notifier=w729) -> (notifier out=w728:refnum<notifier>, current notification=w727:T8)  [unwired: 1 in, 3 out]
              n383 = Unbundle By Name(w727) -> ("Abort If Error"=w715:bool, "XY Stage Move Limit (µm)"=w718:dbl)
              n384 = Array Subset(array=w685, index (row)=0 ("index"), length (row)=2 ("length"), index (col)=2 ("index")) -> (w722:dbl[][])  [unwired: 1 in]
              n385 = Build Array("X Update Scale Factor", "Y Update Scale Factor") -> (w676:dbl[])
              n386 = Array Subset(array=w685, index (row)=0 ("index"), length (row)=2 ("length"), index (col)=3 ("index"), length (col)=1 ("length")) -> (w684:dbl[][])
              n387 = Index Array(array=w722, index (col)=0 ("disabled index (col)")) -> (element=w680:dbl[])  [unwired: 1 in]
              n388 = Index Array(array=w684, index (col)=0 ("disabled index (col)")) -> (element=w682:dbl[])  [unwired: 1 in]
              n389 = Equal?(x=4Pi_Obj_Lock_-_Actions."Move XYZ", y=w695) -> (x = y?=w693:bool)
              n390 = Multiply(x=w680, y=w676) -> (x*y=w679:dbl[])
              n391 = call "Stages Messenger.vi"("Stage Notifier Name"=w699, "Actions"=Stage_Actions."Get Position") -> ("Stage Notifier Name (Dup)"=w698:string, "Positions"=w697:dbl[])  [unwired: 10 in, 2 out]
              n392 = call "4Pi Obj Lock - Rotate Flip XY.vi"("XY Amounts"=w679, "Flip XY"="Flip XY Axis", "Invert X"="Invert X Axis", "Invert Y"="Invert Y Axis") -> ("45° Rotated XY"=w681:dbl[])  [unwired: 11 in]
              n393 = Add(x=w697, y=w681) -> (x+y=w696:dbl[])
              n394 = Select(t=4Pi_Obj_Lock_-_Actions."Move Z" ("x"), s=w693, f=4Pi_Obj_Lock_-_Actions."Update Plots") -> (s? t:f=w690:T6)
              n395 = Add(x=w682, y=w707) -> (x+y=w705:dbl[])
              n396 = Subtract(x=w682, y=w707) -> (x-y=w706:dbl[])
              n397 = Absolute Value(x=w681) -> (abs(x)=w717:dbl[])
              n398 = Greater?(x=w718, y=w717) -> (0:w716:bool[])
              n399 = In Range and Coerce(upper limit=w705, x=w696, lower limit=w706) -> (In Range?=w704:bool[])  [unwired: 1 out]
              n400 = And Array Elements(Boolean array=w716) -> (logical AND=w703:bool)
              n401 = And Array Elements(Boolean array=w704) -> (logical AND=w701:bool)
              n402 = And(x=w703, y=w701) -> (x .and. y?=w702:bool)
              n403 = Not(x=w702) -> (.not. x?=→"Move Limit Error":bool)
              n404 = case shown="True" w702 {
                tunnel: w681 -> [_ w739]
                tunnel: w715 -> [w735 _]
                tunnel: [w733 w736] -> w714
                tunnel: w698 -> [_ w738]
                tunnel: [dbl[] [-1.0, -1.0] ("Positions") w737] -> w712
                tunnel: w690 -> [w731 w736]
                frame False {
                  n405 = Select(t=4Pi_Obj_Lock_-_Actions."Abort" ("x"), s=w735, f=w731) -> (s? t:f=w733:T6)
                }
                frame True {
                  n406 = call "Stages Messenger.vi"("Stage Notifier Name"=w738, "Actions"=Stage_Actions."MVR", "Setpoint"=w739, "Axis"=bool[] [TRUE, TRUE]) -> ("Positions"=w737:dbl[])  [unwired: 8 in, 3 out]
                }
              }
              n407 = Index Array(array=w712, index #1=0 ("index"), index #2=1 ("index")) -> (element #1=→"X Axis Position (µm)":dbl, element #2=→"Y Axis Position (µm)":dbl)
            }
            frame "Move Z" {
              w755 = 2.0 ("y")
              # "Initial Z stage position"
              n408 = Get Notifier Status(notifier=w773) -> (notifier out=w772:refnum<notifier>, current notification=w774:T8)  [unwired: 1 in, 3 out]
              n409 = case shown="False" FALSE {
                tunnel: [w776 w779] -> w767
                tunnel: w749 -> [_ w777]
                frame False {
                  n410 = local read "dz (µm)"() -> (w776:dbl)
                }
                frame True {
                  w778 = 0 ("disabled index (col)")
                  # "Get sx/sy Diff Value"
                  n411 = Array Subset(array=w777, index (row)=2 ("index"), length (row)=1 ("length"), index (col)=2 ("index"), length (col)=1 ("length")) -> (w781:dbl[][])
                  n412 = Index Array(array=w781, index (row)=w778, index (col)=w778) -> (element=w779:dbl)
                }
              }
              n413 = Index Array(array=w749, index (row)=2, index (col)=3 ("disabled index (col)")) -> (element=w746:dbl)
              n414 = Unbundle By Name(w774) -> ("Abort If Error"=w754:bool, "Z Stage Move Limit (µm)"=w759:dbl)
              n415 = Multiply(x=w767, y="Z Update Scale Factor") -> (x*y=w764:dbl)
              n416 = Add(x=w746, y=w755) -> (x+y=w761:dbl)
              n417 = Subtract(x=w746, y=w755) -> (x-y=w760:dbl)
              n418 = call "Stages Messenger.vi"("Stage Notifier Name"=w770, "Actions"=Stage_Actions."Get Position") -> ("Stage Notifier Name (Dup)"=w756:string, "Positions"=w768:dbl[])  [unwired: 10 in, 2 out]
              n419 = Negate(x=w764) -> (-x=w765:dbl)
              n420 = Select(t=w765, s="Invert Z Axis", f=w764) -> (s? t:f=w745:dbl)
              n421 = Index Array(array=w768, index=0) -> (element=w766:dbl)
              n422 = Absolute Value(x=w745) -> (abs(x)=w744:dbl)
              n423 = Add(x=w745, y=w766) -> (x+y=w762:dbl)
              n424 = Greater?(x=w759, y=w744) -> (0:w758:bool)
              n425 = In Range and Coerce(upper limit=w761, x=w762, lower limit=w760) -> (In Range?=w757:bool)  [unwired: 1 out]
              n426 = And(x=w758, y=w757) -> (x .and. y?=w753:bool)
              n427 = Not(x=w753) -> (.not. x?=w752:bool)
              n428 = case shown="True" w753 {
                tunnel: w756 -> [_ w798]
                tunnel: w754 -> [w788 _]
                tunnel: w745 -> [_ w797]
                tunnel: [w787 4Pi_Obj_Lock_-_Actions."Update Plots" ("x")] -> w751
                tunnel: [-1.0 ("Position") w792] -> w750
                frame False {
                  n429 = Select(t=4Pi_Obj_Lock_-_Actions."Abort" ("x"), s=w788, f=4Pi_Obj_Lock_-_Actions."Update Plots") -> (s? t:f=w787:T6)
                }
                frame True {
                  n430 = Build Array(w797) -> (w796:dbl[])
                  n431 = call "Stages Messenger.vi"("Stage Notifier Name"=w798, "Actions"=Stage_Actions."MVR", "Setpoint"=w796, "Axis"=bool[] [TRUE]) -> ("Positions"=w794:dbl[])  [unwired: 8 in, 3 out]
                  n432 = Wait (ms)(milliseconds to wait=u32 50) -> ()  [unwired: 1 out]
                  n433 = Index Array(array=w794, index=0) -> (element=w792:dbl)
                }
              }
              "Z Axis Position (µm)" <- w750
              n434 = local write "Move Limit Error"(w752) -> ()
            }
            frame "Update Plots" {
              # "Current Values"
              # "Target Values"
              n435 = Get Notifier Status(notifier=w840) -> (notifier out=w839:refnum<notifier>, current notification=w841:T8)  [unwired: 1 in, 3 out]
              n436 = Unbundle By Name(w841) -> ("Z Drift Threshold"=w831:dbl, "XY Drift Threshold"=w830:dbl)
              n437 = local read "X Axis Position (µm)"() -> (w825:dbl)
              n438 = local read "Y Axis Position (µm)"() -> (w824:dbl)
              n439 = local read "Z Axis Position (µm)"() -> (w823:dbl)
              n440 = Index Array(array=w820, index (col)=0 ("disabled index (col)")) -> (element=w815:dbl[])  [unwired: 1 in]
              n441 = Index Array(array=w820, index (col)=1 ("disabled index (col)")) -> (element=w816:dbl[])  [unwired: 1 in]
              n442 = Index Array(array=w820, index (col)=3 ("disabled index (col)")) -> (element=w821:dbl[])  [unwired: 1 in]
              n443 = Subtract(x=w816, y=w815) -> (x-y=w814:dbl[])
              n444 = Build Array(w825, w824, w823) -> (w822:dbl[])
              n445 = Index Array(array=w814, index #1=0 ("index"), index #2=1 ("index"), index #3=2 ("index")) -> (element #1=w804:dbl, element #2=w802:dbl, element #3=w806:dbl)
              n446 = Subtract(x=w822, y=w821) -> (x-y=w819:dbl[])
              n447 = Index Array(array=w819, index #1=0 ("index"), index #2=1 ("index"), index #3=2 ("index")) -> (element #1=w818:dbl, element #2=w817:dbl, element #3=w805:dbl)
              n448 = Multiply(x="pixel size (µm)", y=w804) -> (x*y=w803:dbl)
              n449 = Multiply(x="pixel size (µm)", y=w802) -> (x*y=w800:dbl)
              n450 = call "4Pi Obj Lock - 1 Values Organize Plot Data.vi"("Target 01"=0.0, "Value Limit"=w830, "Current 01"=w803, "Stage Pos"=w818) -> ("plot data"=→"X Target and Fit Position (µm)":T2)  [unwired: 11 in]
              n451 = call "4Pi Obj Lock - 1 Values Organize Plot Data.vi"("Target 01"=0.0, "Value Limit"=w830, "Current 01"=w800, "Stage Pos"=w817) -> ("plot data"=→"Y Target and Fit Position (µm)":T2)  [unwired: 11 in]
              n452 = local read "Measured Z (µm)"() -> (w809:dbl)
              n453 = Select(t=w806, s=FALSE, f=w809) -> (s? t:f=w807:dbl)
              n454 = call "4Pi Obj Lock - 1 Values Organize Plot Data.vi"("Target 01"=0.0, "Value Limit"=w831, "Current 01"=w807, "Stage Pos"=w805) -> ("plot data"=→"Z Target and Fit Value (µm)":T2)  [unwired: 11 in]
            }
            frame "Delay" {
              n455 = Get Notifier Status(notifier=w849) -> (notifier out=w847:refnum<notifier>, current notification=w850:T8)  [unwired: 1 in, 3 out]
              n456 = Unbundle By Name(w850) -> ("Update Delay (ms)"=w846:i32)
              n457 = while {
                tunnel: w847 -> [w862]
                tunnel: w846 -> [w859]
                tunnel: [w855] -> w845
                i -> [w860]
                stop <- w853 stop-if-true
                n458 = Get Notifier Status(notifier=w862) -> (notifier out=w855:refnum<notifier>, current notification=w858:T8)  [unwired: 1 in, 3 out]
                n459 = Greater Or Equal?(x=w860, y=w859) -> (x >= y?=w854:bool)
                n460 = Wait (ms)(milliseconds to wait=u32 1) -> ()  [unwired: 1 out]
                n461 = Unbundle By Name(w858) -> ("Actions"=w857:T6)
                n462 = Equal?(x=w857, y=4Pi_Obj_Lock_-_Actions."Abort") -> (x = y?=w852:bool)
                n463 = Or(x=w852, y=w854) -> (x .or. y?=w853:bool)
              }
            }
            frame "Abort" {
              w866 = 0.0 ("Target X Position (px)")
              n464 = Get Notifier Status(notifier=w872) -> (notifier out=w876:refnum<notifier>, current notification=w875:T8)  [unwired: 1 in, 3 out]
              n465 = call "Camera Messenger.vi"("Notifier Name"=w864, "General Camera Actions"=Generic_Camera_Actions."Abort") -> ()  [unwired: 8 in, 6 out]
              n466 = Bundle By Name(cluster=w875, "Running?"=FALSE, "Actions"=4Pi_Obj_Lock_-_Actions."Exit Loop") -> (w873:T8)
              n467 = Send Notification(notification=w873, notifier=w876) -> (notifier out=w871:refnum<notifier>)  [unwired: 1 in, 1 out]
              n468 = local write "Start Lock"(FALSE ("Start Lock")) -> ()
              n469 = local write "Measured X Position (px)"(w866) -> ()
              n470 = local write "Measured Y Position (px)"(w866) -> ()
              n471 = local write "Target X Position (px)"(w866) -> ()
              n472 = local write "Target Y Position (px)"(w866) -> ()
              n473 = local write "Measured sx/sy"(w866) -> ()
              n474 = local write "Target sx/sy"(w866) -> ()
            }
            frame "Exit Loop" {
            }
            frame "Quit" {
              n475 = Get Notifier Status(notifier=w882) -> (notifier out=w881:refnum<notifier>, current notification=w889:T8)  [unwired: 1 in, 3 out]
              n476 = Unbundle By Name(w889) -> ("Ref Stack (SGL)"=w888:T9[], "Cur Image (SGL)"=w887:T9, "Tmp Image FFT (CSG)"=w886:T9[], "CC Image (SGL)"=w885:T9, "Ref FFT Stack (CSG)"=w883:T9[])
              n477 = Release Notifier(notifier=w881, force destroy? (F)=TRUE) -> ()  [unwired: 1 in, 3 out]
              n478 = Build Array (concatenate)(w888, w887, w886, w885, w883) -> (w884:T9[])
              n479 = for {
                tunnel: w884 -> [w894] mode=indexing
                n480 = call "IMAQ Dispose"("Image"=w894) -> ()  [unwired: 5 in, 1 out]
              }
            }
          }
          n481 = Get Notifier Status(notifier=w231) -> (current notification=w230:T8, error out=w225:errorcluster)  [unwired: 1 in, 3 out]
          n482 = Unbundle By Name(w230) -> ("Actions"=w229:T6)
          n483 = Unbundle By Name(w225) -> ("status"=w223:bool)
          n484 = Equal?(x=w228, y=w229) -> (x = y?=w224:bool)
          n485 = Or(x=w224, y=w223) -> (x .or. y?=w222:bool)
          n486 = Select(t=w228, s=w222, f=w227) -> (s? t:f=w226:T6)
        }
      }
      n487 = local write "Quit"(w205) -> ()
    }
    frame Error {
    }
  }
  n488 = control-ref of="This VI"() -> (w84:refnum<vi>)
  n489 = property class="VI"(reference=w84) -> (reference out=w93:refnum<vi>, "Panel"=w85:refnum<vi>)  [unwired: 1 in, 1 out]
  n490 = property class="Pnl"(reference=w85) -> ("Decos[]"=w83:refnum<vi>[], "Panes[]"=w89:refnum<vi>[])  [unwired: 1 in, 2 out]
  n491 = Array Size(array=w83) -> (size(s)=w81:i32)
  n492 = Decrement(x=w81) -> (x-1=w82:i32)
  n493 = Index Array(array=w89, index=0) -> (element=w88:refnum<vi>)
  n494 = Index Array(array=w83, index=w82) -> (element=w91:refnum<vi>)
  n495 = property class="VI"(reference=w93) -> (reference out=w95:refnum<vi>, "Front Panel.PanelBounds"=w96:T22)  [unwired: 1 in, 1 out]
  n496 = property class="Decor"(reference=w91) -> ("Bounds"=w94:T23)  [unwired: 1 in, 2 out]
  n497 = property class="Pane"(reference=w88, "Origin"=T11 {"Horizontal"=0, "Vertical"=0}, "HorizScrollbarVisibility"=w92, "VertScrollbarVisibility"=w92) -> ()  [unwired: 1 in, 2 out]
  n498 = Unbundle By Name(w94) -> ("Width"=w99:u32, "Height"=w102:u32)
  n499 = control-ref of="Quit"() -> (w86:refnum<vi>)
  n500 = To Word Integer(number=w99) -> (16bit integer=w101:i16)
  n501 = To Word Integer(number=w102) -> ()  [unwired: 1 out]
  n502 = property class="Bool (strict)"(reference=w86) -> ("Height"=w104:u32, "Top"=w105:i32)  [unwired: 1 in, 2 out]
  n503 = Unbundle By Name(w96) -> ("Left"=w98:i16, "Top"=w109:i16)
  n504 = To Word Integer(number=w104) -> (16bit integer=w107:i16)
  n505 = To Word Integer(number=w105) -> (16bit integer=w108:i16)
  n506 = Add(x=w98, y=w101) -> (x+y=w100:i16)
  n507 = Compound Arithmetic op=ADD(w109, w107, w108, i16 12 ("y")) -> (w103:i16)
  n508 = Bundle By Name(cluster=w96, "Right"=w100, "Bottom"=w103) -> (w97:T22)
  n509 = property class="VI"(reference=w95, "Front Panel.PanelBounds"=w97) -> ()  [unwired: 1 in, 2 out]
